vi "PositionSave_coMD.vi"() -> ()   [LabVIEW 2012]
doc: "SciScan 1.2 160622\n<b>Description</b>\n-------------\nThis is the Main VI for the Position Save Module and has a UI.\n\nThe module has a dependency with the main Sci-Scan software as it listens for events using the GFG."
uses:
  Custom Control and Typedefs/ChannelSelector_for_PosSave.ctl
  Custom Controls/PositionSaveMod.ctl
  Custom Control and Typedefs/Overlay Control.ctl
  SubVIs/PositionSaveFGVCommands.ctl
  Custom Control and Typedefs/UI Controls Refnum.ctl
  <vilib>/vision/Image Controls.llb/IMAQ Image.ctl
  Custom Control and Typedefs/ImageCluster.ctl
  SubVIs/Chnl_2_tab_Commands.ctl
  SubVIs/Image Validity FGV_Commands.ctl
  Custom Controls/MAIN Image panel tab Control type def.ctl
  CommonResource VIs/UI Control and Indicator properties_Commands.ctl
  CommonResource VIs/FormatTableStyle_Commands.ctl
  Custom Control and Typedefs/PositionData.ctl
  SubVIs/ImageIO_commands.ctl
  GFG/GFG library.lvlib
panel:
  in  "no of grid lines 2":dbl(slide)=2.0 caption="Grid" min=0.0 step=1.0 scale=0.0..20.0
  in  "FOCUS2":bool
  in  "Overlay Controls":T1={"auto scale\n      Red "=TRUE, "Min Max Saved (Green)"={0.0, 2047.0}, "auto scale\n      Blue"=TRUE, "Min Max Saved (Red)"={0.0, 2047.0}} {"Min Max Saved (Red)" scale=0.0..2047.0; "Min Max Saved (Green)" scale=0.0..2047.0}
  in  "Hide":T2
  in  "Copy Button":bool
  out "File Path":path
  in  "Overlay":bool
  in  "Table Navigation Cluster":T3
  in  "Vert_Cluster":T4
  in  "Big_Table":string[][](table)
  in  "Notes_Table":string[][](table)
  in  "Source":T5
  in  "step.size.z 2":u16(ring)=6 items=["  1"=1, "  2"=2, "  5"=5, " 10"=10, " 20"=20, " 50"=50, "100"=100]
  in  "Stage Stop 2":bool
  in  "Z UP 2":bool
  in  "Z DOWN 2":bool
  out "String 26":string
  in  "step.size.xy 2":u16(ring)=6 items=["  1"=1, "  2"=2, "  5"=5, " 10"=10, " 20"=20, " 50"=50, "100"=100]
  in  "Y UP 2":bool
  in  "X LEFT 2":bool
  in  "Y DOWN 2":bool
  in  "X RIGHT 2":bool
  out "String 25":string
  in  "setY 2":dbl caption="Z-Stepper" format="%#.1f"
  in  "setX 2":dbl caption="Z-Stepper" format="%#.1f"
  in  "setZ 2":dbl caption="set" format="%#.1f"
  out "String 24":string
  out "posZ 2":dbl caption="actual" format="%#.1f"
  out "posX 2":dbl caption="Z-Stepper" format="%#.1f"
  out "posY 2":dbl caption="Z-Stepper" format="%#.1f"
  out "String 23":string
  in  "Hor_Cluster":T6
  out "XY Graph":cluster{dbl[], dbl[]}[](graph)
  out "Saved Image":T7(plugin-control)
  out "Current Image":T7(plugin-control)
  # "abs  pos."
  # "x"
  # "y"
  # "z"
  # "pos."
  # "x"
  # "y"
  # "z"
  # "Red (Current Image)"
  # "Blue (Saved Image)"
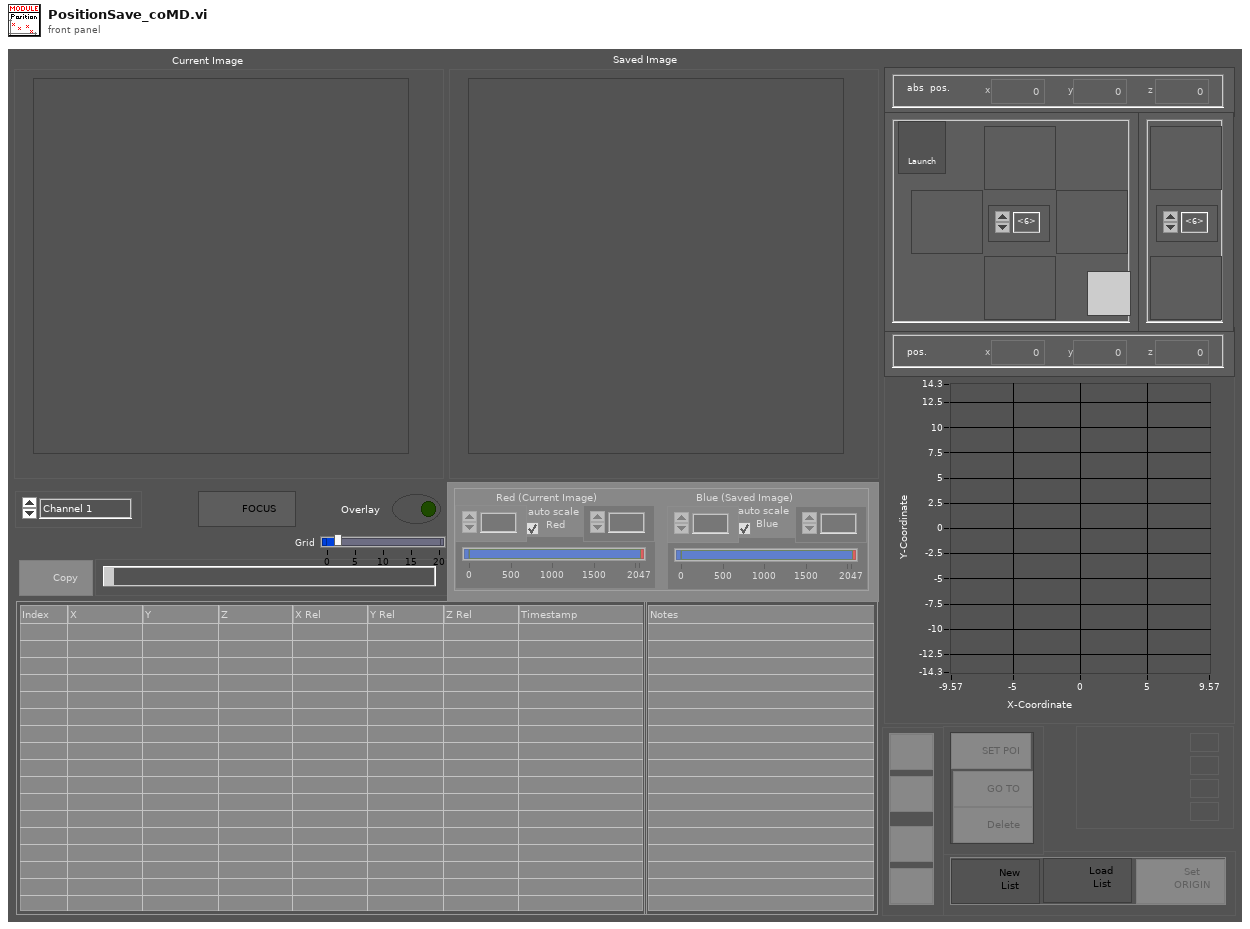
[diagram p1: front panel]
types:
  T1 = typedef "Overlay Control.ctl" = cluster{"auto scale\n      Red ":bool, "Min Max Saved (Green)":cluster{dbl, dbl}, "auto scale\n      Blue":bool, "Min Max Saved (Red)":cluster{dbl, dbl}}
  T2 = typedef "PositionSaveMod.ctl" = bool
  T3 = cluster{"Table Index Up":bool, "Table Index Up-End":bool, "Table Index Down":bool, "Table Index Down-End":bool}
  T4 = cluster{"Delete item":bool, "SET POI":bool, "GO TO":bool}
  T5 = typedef "ChannelSelector_for_PosSave.ctl" = enum16{"Channel 1", "Channel 2", "Channel 3", "Channel 4"}
  T6 = cluster{"New List":bool, "Load List":bool, "Set new Origin":bool}
  T7 = typedef "IMAQ Image.ctl" = refnum<image>
  T8 = typedef "Image Type" = u32
  T9 = typedef "UI Controls Refnum.ctl" = cluster{"GO TO":refnum<vi>, "Load List":refnum<vi>, "Big Table":refnum<vi>, "Notes Table":refnum<vi>, "New List":refnum<vi>, "Delete Item":refnum<vi>, "Set New Origin":refnum<vi>, "Set POI":refnum<vi>, "Saved Image":refnum<vi>, "Current Image":refnum<vi>, "step.size.xy 2":refnum<vi>, "step.size.z 2":refnum<vi>, "Source":refnum<vi>, "Table Up-End":refnum<vi>, "Table Up":refnum<vi>, "Table Down":refnum<vi>, "Table Down-End":refnum<vi>, "Copy Button":refnum<vi>, "Hide":refnum<vi>, "Overlay Controls":refnum<vi>, "Overlay":refnum<vi>, "XYGraph":refnum<vi>, "FOCUS2":refnum<vi>}
  T10 = typedef "PositionSaveFGVCommands.ctl" = enum16{"Initialize", "NewList", "LoadList", "CopyList", "DeleteSelected", "SetPosition", "SetNewOrigin", "UpdateEntireTable", "GetPosition", "Shutdown and Cleanup"}
  T11 = enum8{"Enabled", "Disabled", "Disabled and Grayed Out"}
  T12 = typedef "ImageCluster.ctl" = cluster{"CurrentImage":T7, "SavedImage":T7}
  T13 = enum32{"Invalid", "Standard", "Closed", "Hidden", "Minimized", "Maximized"}
  T14 = typedef "Image Validity FGV_Commands.ctl" = enum16{"Set validity status", "Get Validity status"}
  T15 = typedef "Chnl_2_tab_Commands.ctl" = enum16{"ChannelToTab", "TabToChannel"}
  T16 = typedef "MAIN Image panel tab Control type def.ctl" = enum32{"Channel 1", "Channel 2", "Channel 3", "Channel 4", "all channels", "RGB overlay", "ROI", "arbitrary line scan"}
  T17 = typedef "UI Control and Indicator properties_Commands.ctl" = enum16{"Enable", "Disable", "Disable and Grey", "Make Visible", "Make Invisible"}
  T18 = cluster{"moveXabs":dbl, "moveYabs":dbl, "moveZabs":dbl}
  T19 = typedef "FormatTableStyle_Commands.ctl" = enum16{"Colour Row", "Uncolour Row", "Bold Row", "Clear table", "UpdateVisibleRows", "Set Row Height", "Enabled Row style", "Disabled Row Style"}
  T20 = typedef "PositionData.ctl" = cluster{"X":dbl, "Y":dbl, "Z":dbl, "Base Path":path}
  T21 = typedef "ImageIO_commands.ctl" = enum16{"ReadImage", "WriteImage"}
  T22 = cluster{"WaveformChartRef":refnum<vi>, "DigitalRef":refnum<vi>, "ArrayRef":refnum<vi>, "TabControlRef":refnum<vi>, "EnumRef":refnum<vi>, "RingRef":refnum<vi>, "BooleanRef":refnum<vi>, "KnobRef":refnum<vi>, "SlideRef":refnum<vi>, "PathRef":refnum<vi>, "StringRef":refnum<vi>, "ComboBox":refnum<vi>, "WaveformGraphRef":refnum<vi>}
  T23 = typedef "LVRowAndColumnTypeDef.ctl" = cluster{"Row":i32, "Column":i32}
  T24 = typedef "eventvkey.ctl" = enum16{"ASCII", "Enter", "Return", "Shift", "Ctrl", "Alt", "Cmd", "Opt", "Caps", "NumLock", "Clear", "Break", "Up", "Down", "Left", "Right", "Insert", "Delete", "Home", "End", "PageUp", "PageDown", "Escape", "Help", "Pause", "ScrollLock", "F1", "F2", "F3", "F4", "F5", "F6", "F7", "F8", "F9", "F10", "F11", "F12", "F13", "F14", "F15", "F16", "F17", "F18", "F19", "F20", "F21", "F22", "F23", "F24", "Play", "VolumeUp", "VolumeDown", "Mute", "Two Byte Char"}
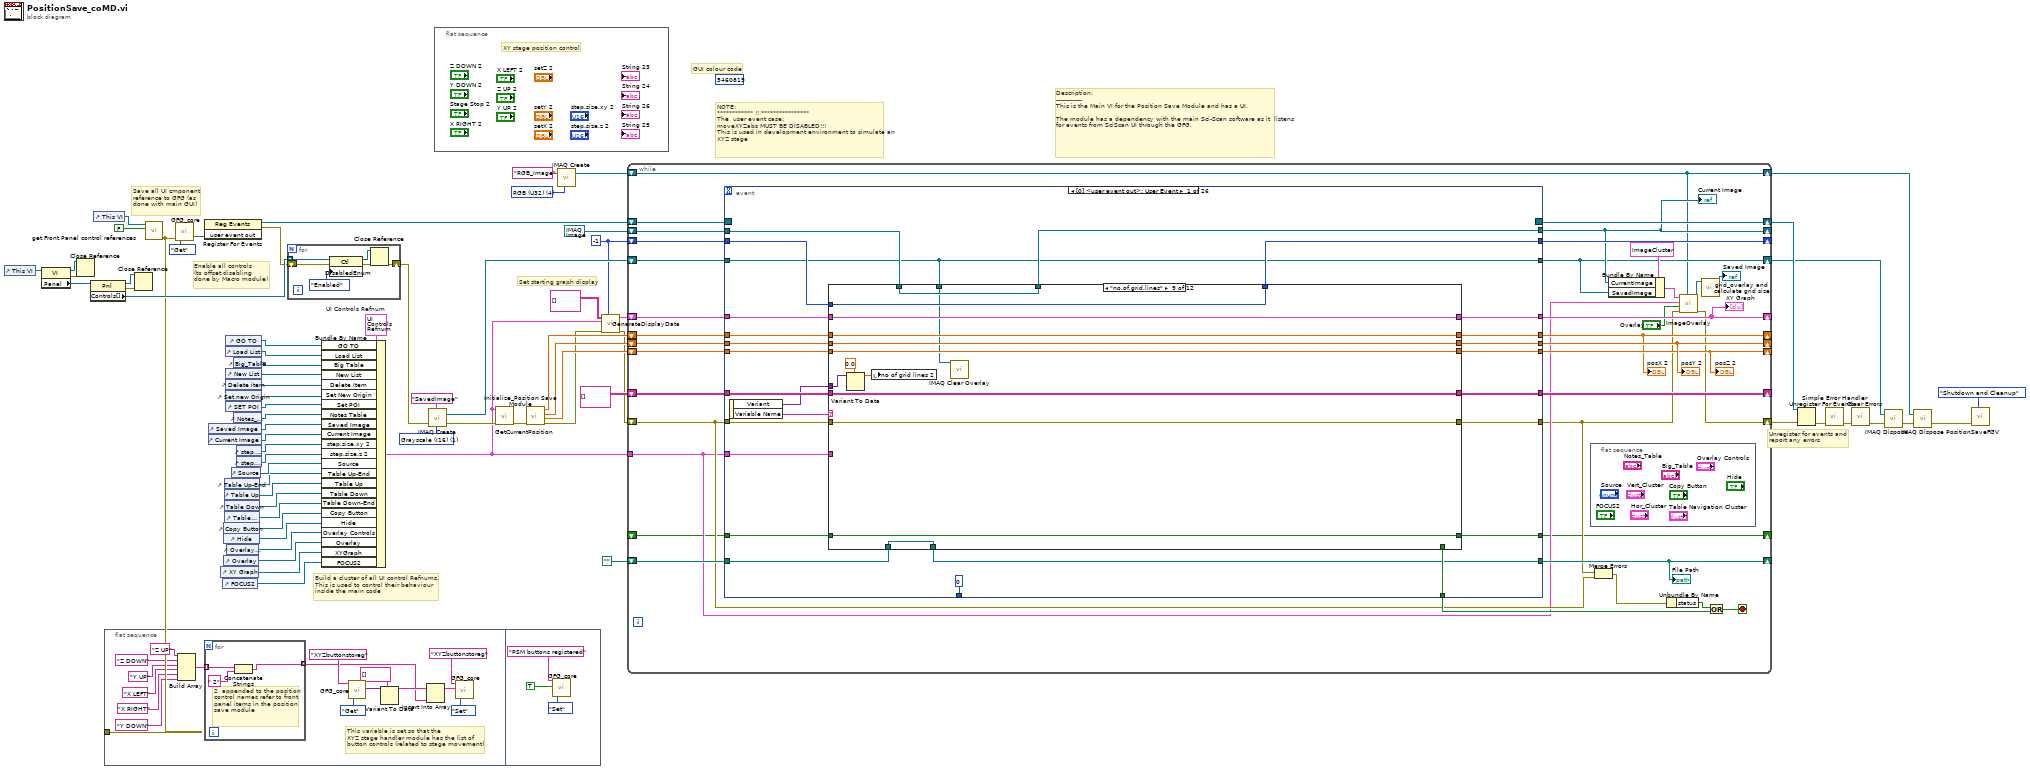
[diagram p0: block diagram]
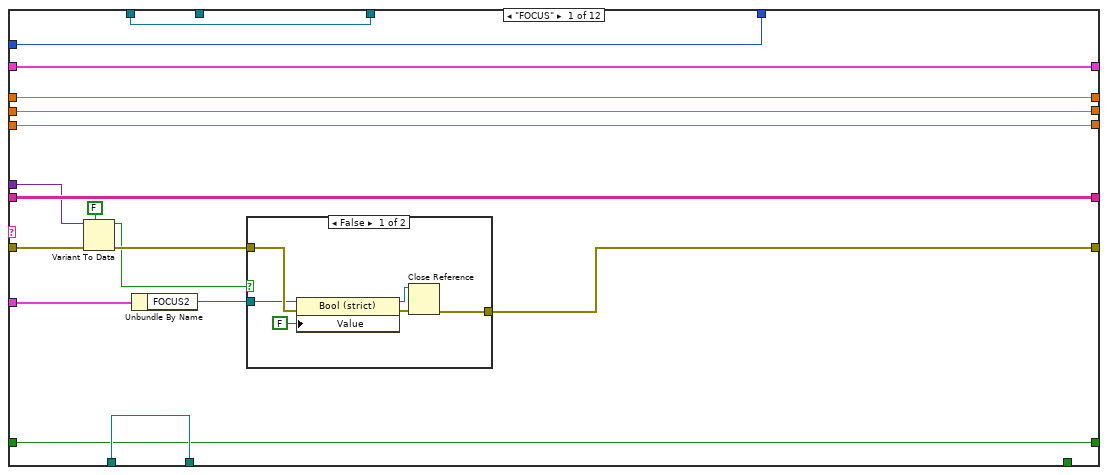
[diagram p2: hidden frame]
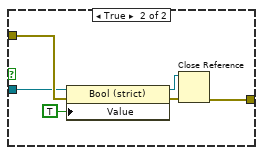
[diagram p3: hidden frame]
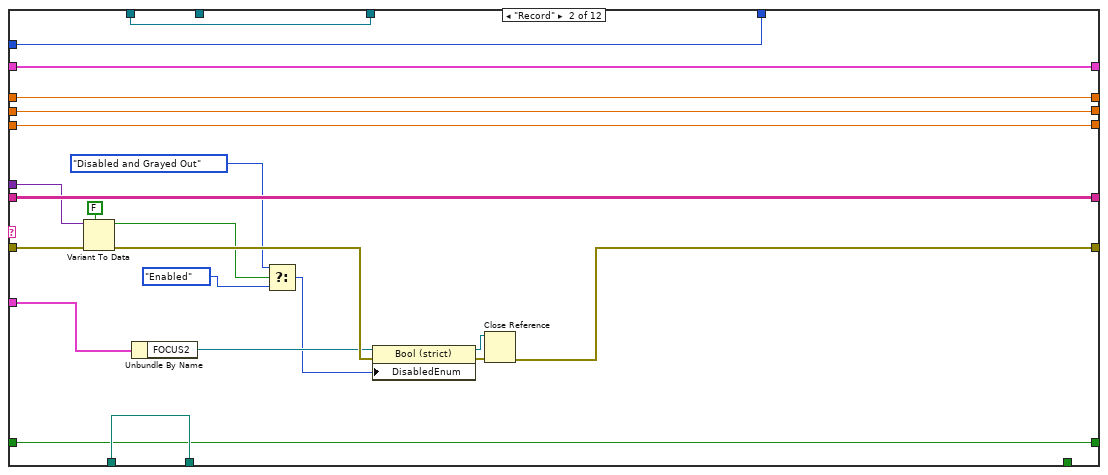
[diagram p4: hidden frame]
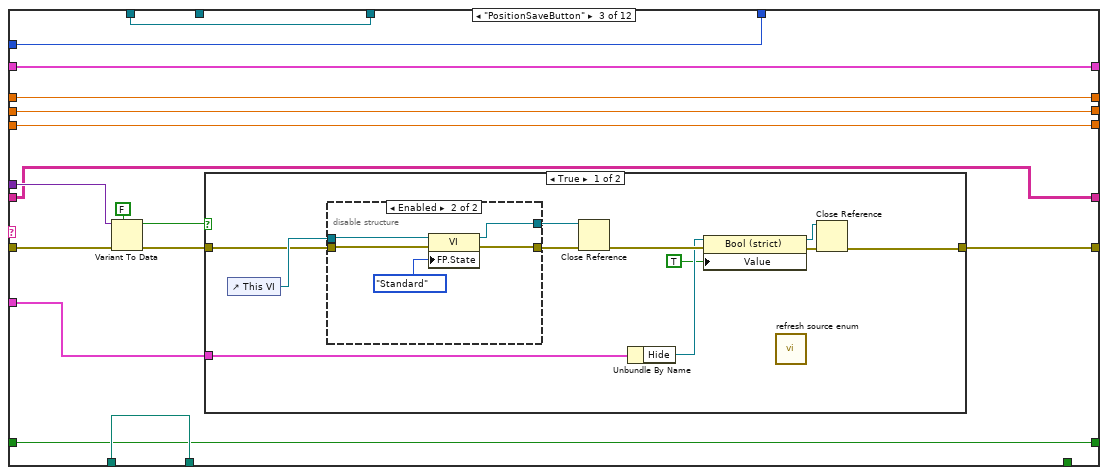
[diagram p5: hidden frame]
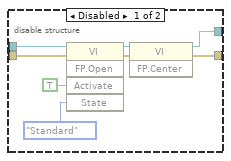
[diagram p6: hidden frame]
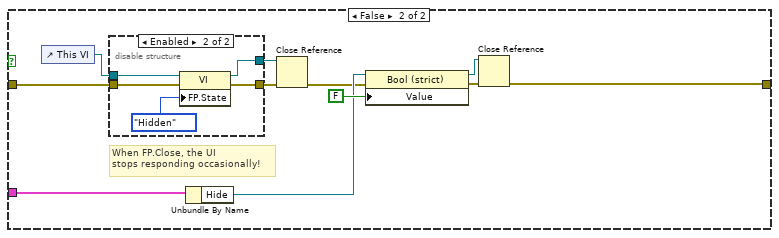
[diagram p7: hidden frame]
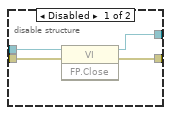
[diagram p8: hidden frame]
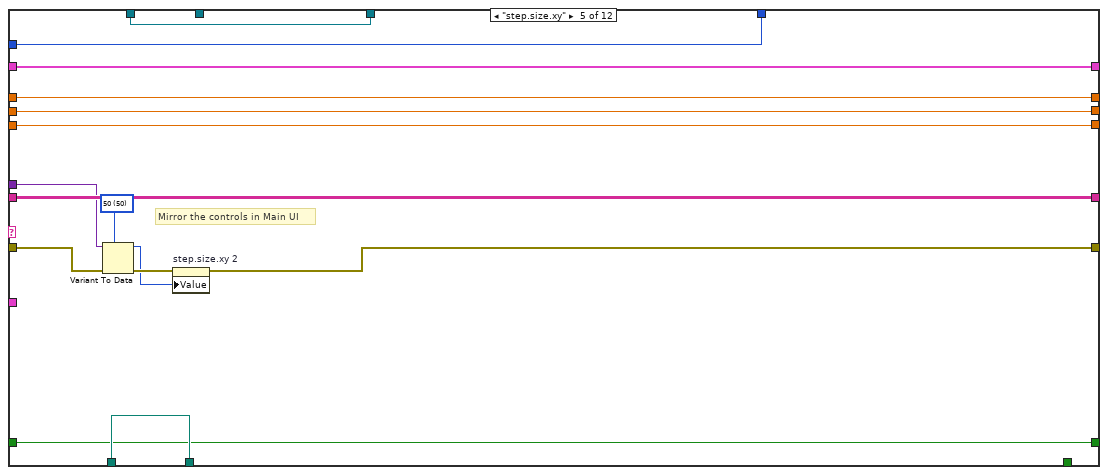
[diagram p10: hidden frame]
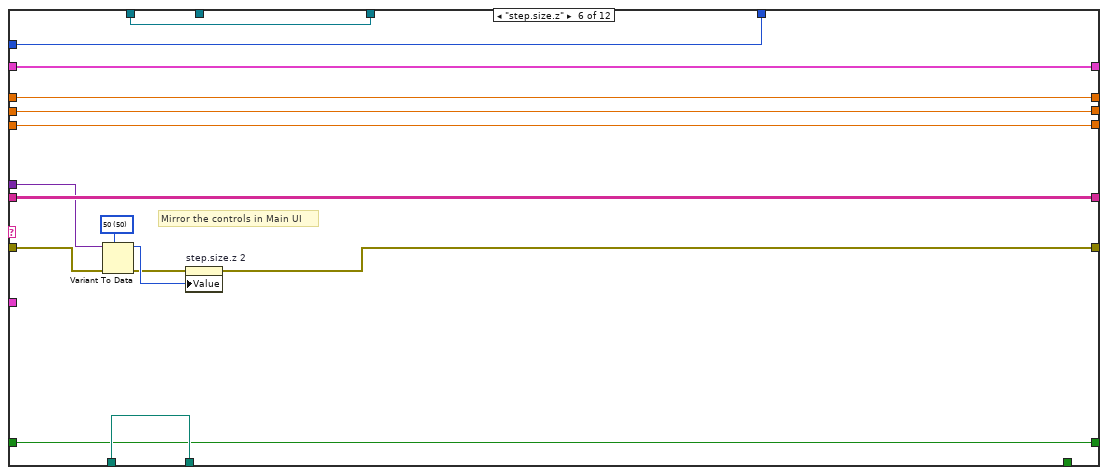
[diagram p11: hidden frame]
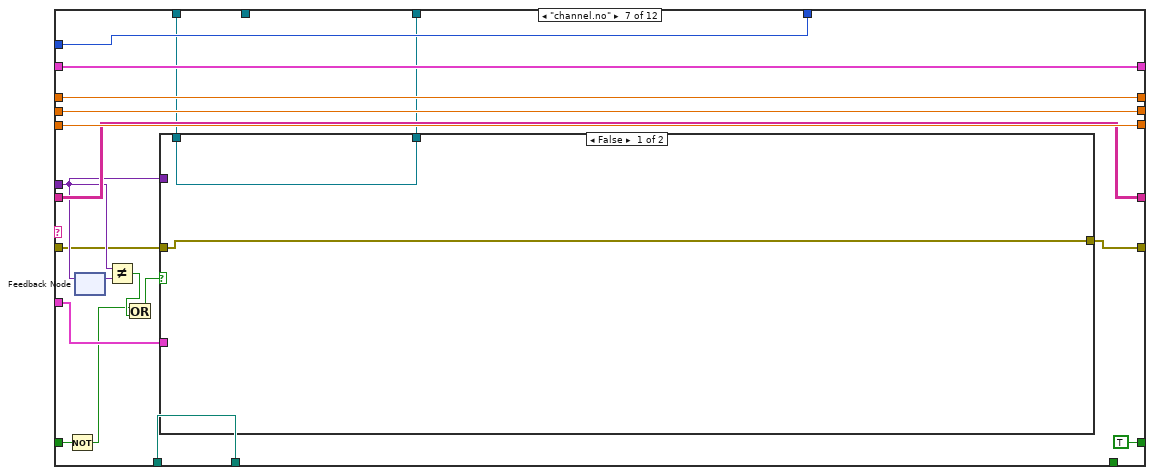
[diagram p12: hidden frame]
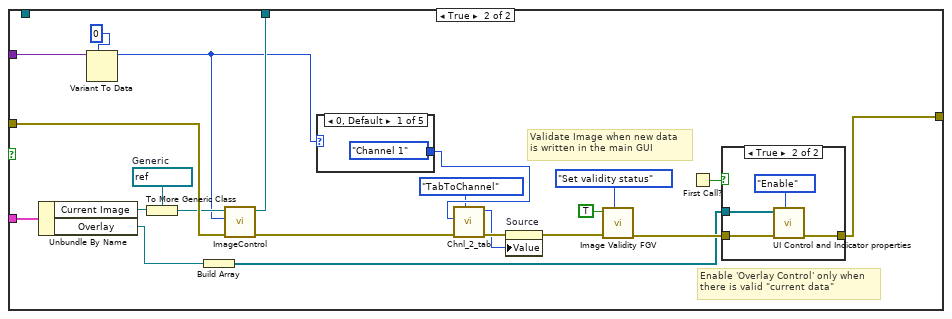
[diagram p13: hidden frame]
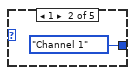
[diagram p14: hidden frame]
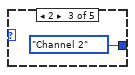
[diagram p15: hidden frame]
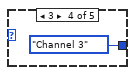
[diagram p16: hidden frame]
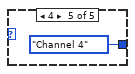
[diagram p17: hidden frame]
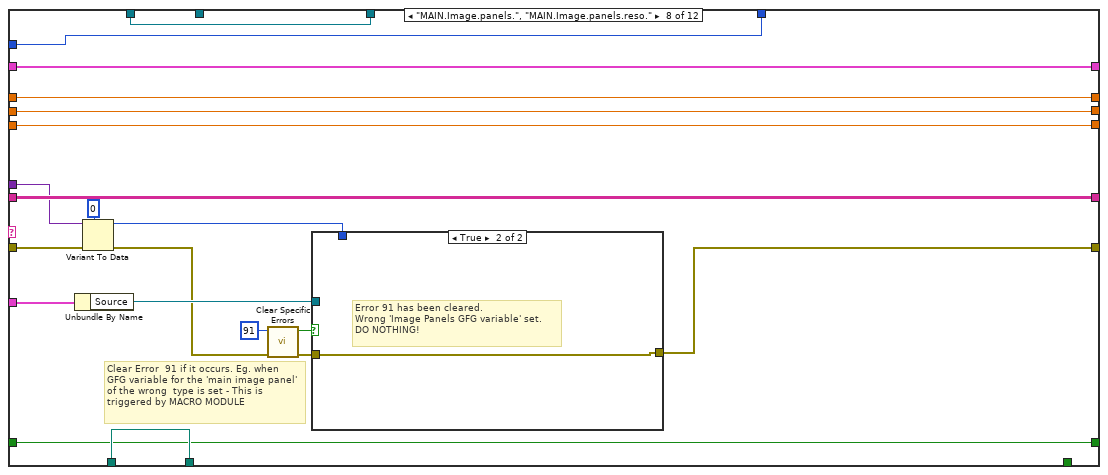
[diagram p19: hidden frame]
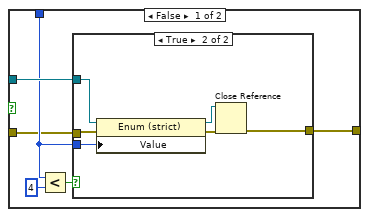
[diagram p20: hidden frame]
diagram:
  w26 = T8 4 items=["Grayscale (U8)", "Grayscale (I16)", "Grayscale (SGL)", "Complex (CSG)", "RGB (U32)", "HSL (U32)", "RGB (U64)", "Grayscale (U16)"] ("Image Type")
  w37 = T8 1 items=["Grayscale (U8)", "Grayscale (I16)", "Grayscale (SGL)", "Complex (CSG)", "RGB (U32)", "HSL (U32)", "RGB (U64)", "Grayscale (U16)"] ("Image Type")
  (unwired) u32 5460819 ("Active Cell:Cell Background Color")
  w18 = -1
  w61 = T9 {"GO TO"=refnum, "Load List"=refnum, "Big Table"=refnum, "Notes Table"=refnum, "New List"=refnum, "Delete Item"=refnum, "Set New Origin"=refnum, "Set POI"=refnum, "Saved Image"=refnum, "Current Image"=refnum, "step.size.xy 2"=refnum, "step.size.z 2"=refnum, "Source"=refnum, "Table Up-End"=refnum, "Table Up"=refnum, "Table Down"=refnum, "Table Down-End"=refnum, "Copy Button"=refnum, "Hide"=refnum, "Overlay Controls"=refnum, "Overlay"=refnum, "XYGraph"=refnum, "FOCUS2"=refnum}  # UI Controls Refnum
  # "Enable all controls\n(to offset disabling \ndone by Macro module)"
  # "Set starting graph display"
  # "GUI colour code"
  # "Save all UI cmponent reference to GFG (as done with main GUI)"
  # "NOTE:\n************ !! ****************\nThe  user event case:\nmoveXYZabs MUST BE DISABLED!!!\nThis is used in development environment to simulate an XYZ stage"
  # "Build a cluster of all UI control Refnums.\nThis is used to control their behaviour \ninside the main code"
  # "Unregister for events and \nreport any errors"
  # "Description:\n-------------\nThis is the Main VI for the Position Save Module and has a UI.\n\nThe module has a dependency with the main Sci-Scan software as it  listens for events from SciScan UI through the GFG."
  n1 = control-ref of="This VI"() -> (w10:refnum<vi>)
  n2 = property class="VI"(reference=w10) -> (reference out=w7:refnum<vi>, error out=w8:errorcluster, "Panel"=w9:refnum<vi>)  [unwired: 1 in]
  n3 = Close Reference(reference=w7, error in (no error)=w8) -> ()  [unwired: 1 out]
  n4 = property class="Pnl"(reference=w9) -> (reference out=w5:refnum<vi>, error out=w6:errorcluster, "Controls[]"=w4:refnum<vi>[])  [unwired: 1 in]
  n5 = control-ref of="This VI"() -> (w54:refnum<vi>)
  n6 = flat-sequence {
    tunnel: w1 -> [_]
    frame #0 {
      # "This variable is set so that the \nXYZ stage handler module has the list of\nbutton controls (related to stage movement)"
      n7 = Build Array("Z UP" ("Variable Name in"), "Z DOWN" ("Variable Name in"), "Y UP" ("Variable Name in"), "X LEFT" ("Variable Name in"), "X RIGHT" ("Variable Name in"), "Y DOWN" ("Variable Name in")) -> (w79:string[])
      n8 = for {
        tunnel: w79 -> [w88] mode=indexing
        tunnel: [w86] -> w70 mode=indexing
        # "2  appended to the position control names refer to front panel items in the position save module"
        n9 = Concatenate Strings(w88, " 2" ("string")) -> (w86:string)
      }
      n10 = call "GFG_core.vi"("Variable Name in"="XYZbuttonstoreg", "Action"=enum16{"Init", "Set", "Get"}."Get") -> ("Variant Out"=w73:variant)  [unwired: 11 in, 6 out]
      n11 = Variant To Data(type=string[] [], Variant=w73) -> (data=w71:string[])  [unwired: 1 in, 1 out]
      n12 = Insert Into Array(array=w71, new element=w70) -> (w72:string[])  [unwired: 1 in]
      n13 = call "GFG_core.vi"("Variable Name in"="XYZbuttonstoreg", "Variant in"=w72, "Action"=enum16{"Init", "Set", "Get"}."Set") -> ()  [unwired: 10 in, 7 out]
    }
    frame #1 {
      n14 = call "GFG_core.vi"("Variable Name in"="PSM buttons registered", "Variant in"=TRUE, "Action"=enum16{"Init", "Set", "Get"}."Set") -> ()  [unwired: 10 in, 7 out]
    }
  }
  n15 = Close Reference(reference=w5, error in (no error)=w6) -> ()  [unwired: 1 out]
  n16 = call "get Front Panel control references.vi"("Signalling (Default: T)"=FALSE, "Main VI"=w54) -> ("error out"=w1:errorcluster)  [unwired: 9 in]
  n17 = call "GFG_core.vi"("error in (no error)"=w1, "Action"=enum16{"Init", "Set", "Get"}."Get") -> ("user event out"=w67:refnum<user-event>)  [unwired: 11 in, 6 out]
  n18 = register-events(w67) -> (reference out=w68:refnum<event-registration>, error out=w3:errorcluster)  [unwired: 2 in]
  n19 = control-ref of="Saved Image"() -> (w50:refnum<vi>)
  n20 = control-ref of="Current Image"() -> (w49:refnum<vi>)
  n21 = control-ref of="XY Graph"() -> (w22:refnum<vi>)
  n22 = control-ref of="FOCUS2"() -> (w17:refnum<vi>)
  n23 = control-ref of="Overlay"() -> (w23:refnum<vi>)
  n24 = control-ref of="Copy Button"() -> (w35:refnum<vi>)
  n25 = control-ref of="Hide"() -> (w31:refnum<vi>)
  n26 = control-ref of="Table Up-End"() -> (w44:refnum<vi>)
  n27 = control-ref of="Table Up"() -> (w43:refnum<vi>)
  n28 = control-ref of="Table Down"() -> (w42:refnum<vi>)
  n29 = control-ref of="Table Down-End"() -> (w41:refnum<vi>)
  n30 = control-ref of="GO TO"() -> (w60:refnum<vi>)
  n31 = control-ref of="Load List"() -> (w59:refnum<vi>)
  n32 = control-ref of="New List"() -> (w58:refnum<vi>)
  n33 = control-ref of="Delete item"() -> (w57:refnum<vi>)
  n34 = control-ref of="Set new Origin"() -> (w56:refnum<vi>)
  n35 = control-ref of="SET POI"() -> (w55:refnum<vi>)
  n36 = control-ref of="Overlay Controls"() -> (w28:refnum<vi>)
  n37 = control-ref of="Source"() -> (w46:refnum<vi>)
  n38 = control-ref of="Big_Table"() -> (w40:refnum<vi>)
  n39 = control-ref of="Notes_Table"() -> (w52:refnum<vi>)
  n40 = control-ref of="step.size.xy 2"() -> (w48:refnum<vi>)
  n41 = control-ref of="step.size.z 2"() -> (w47:refnum<vi>)
  n42 = for {
    tunnel: w4 -> [w97] mode=indexing
    shift-right: [w93] -> w2
    shift-left: w3 -> [w92]
    n43 = property class="Ctl"(reference=w97, error in=w92, "DisabledEnum"=T11."Enabled" ("Disabled")) -> (reference out=w94:refnum<vi>, error out=w95:errorcluster)
    n44 = Close Reference(reference=w94, error in (no error)=w95) -> (error out=w93:errorcluster)
  }
  n45 = Bundle By Name(cluster=w61, "GO TO"=w60, "Load List"=w59, "Big Table"=w40, "New List"=w58, "Delete Item"=w57, "Set New Origin"=w56, "Set POI"=w55, "Notes Table"=w52, "Saved Image"=w50, "Current Image"=w49, "step.size.xy 2"=w48, "step.size.z 2"=w47, "Source"=w46, "Table Up-End"=w44, "Table Up"=w43, "Table Down"=w42, "Table Down-End"=w41, "Copy Button"=w35, "Hide"=w31, "Overlay Controls"=w28, "Overlay"=w23, "XYGraph"=w22, "FOCUS2"=w17) -> (w21:T9)
  n46 = call "IMAQ Create"("Image Name"="SavedImage", "Image Type"=w37, "error in (no error)"=w2) -> ("New Image"=w36:T7, "error out"=w38:errorcluster)  [unwired: 2 in]
  n47 = flat-sequence {
    frame #0 {
      # "XY stage position control"
    }
  }
  n48 = call "Initialize_Position Save Module.vi"("Error In"=w38, "UI Controls Refnum"=w21) -> ("Error Out"=w45:errorcluster)  [unwired: 9 in]
  n49 = call "GetCurrentPosition.vi"("Error In"=w45) -> ("Error Out"=w20:errorcluster, "Z"=w64:dbl, "Y"=w65:dbl, "X"=w66:dbl)  [unwired: 7 in]
  n50 = call "IMAQ Create"("Image Name"="RGB_Image", "Image Type"=w26) -> ("New Image"=w25:T7)  [unwired: 3 in, 1 out]
  n51 = call "GenerateDisplayData.vi"("Index"=w18, "Error In"=w20, "UI Controls Refnum"=w21, "2D Data IN"=string[][] []) -> ("Error Out"=w19:errorcluster, "Plot Data OUT"=w29:cluster{dbl[], dbl[]}[])  [unwired: 4 in, 2 out]
  n52 = while {
    shift-right: [w102] -> w33
    shift-left: w19 -> [w112]
    shift-right: [w129] -> w62
    shift-left: w68 -> [w130]
    shift-right: [w114] -> _
    shift-left: w66 -> [w128]
    shift-right: [w123] -> _
    shift-left: w65 -> [w127]
    shift-right: [w122] -> _
    shift-left: w64 -> [w126]
    shift-right: [w113] -> _
    shift-left: w29 -> [w125]
    shift-right: [w120] -> _
    shift-left: string[][] [] ("Formatted Table Data") -> [w124]
    tunnel: w21 -> [w110]
    shift-right: [w108] -> _
    shift-left: T7 refnum ("Saved Image OUT") -> [w121]
    shift-right: [w118] -> _
    shift-left: w18 -> [w119]
    shift-right: [w107] -> w13
    shift-left: w36 -> [w117]
    shift-right: [w115] -> _
    shift-left: path "" -> [w116]
    shift-right: [w105] -> w12
    shift-left: w25 -> [w105]
    shift-right: [w101] -> _
    shift-left: _ -> [w100]
    stop <- w131 stop-if-true
    n53 = event shown="[0] <user event out>: User Event" {
      selector: w130 -> [_ _ _ _ w596 w676 w743 w869 w951 w1060 _ _ w1268 w1299 _ _ _ _ _ _ _ _ _ _ _ _]
      dyn-events: [_ _ _ _ w589 w670 w738 w867 w946 w1056 _ _ w1263 w1291 _ _ _ _ _ _ _ _ _ _ _ _] -> w129
      timeout: _ -> [_ _ _ _ _ _ _ _ _ _ _ _ _ _ _ _ _ _ _ _ _ _ _ _ _ _]
      tunnel: [w159 _ _ _ _ _ _ _ _ _ _ _ _ _ _ _ _ _ _ _ _ _ _ _ FALSE _] -> w133
      tunnel: w128 -> [w155 w543 w559 w581 w588 w669 w771 w866 w945 w1054 w1183 w1235 w1262 w1294 w1372 w1421 w1471 w1516 w1564 w1595 w1615 w1635 w1696 w1713 w1720 w1766]
      tunnel: w127 -> [w154 w542 w558 w580 w587 w668 w770 w865 w944 w1053 w1182 w1234 w1261 w1293 w1371 w1420 w1470 w1515 w1563 w1594 w1614 w1634 w1695 w1712 w1719 w1765]
      tunnel: w126 -> [w153 w541 w557 w579 w586 w667 w760 w864 w943 w1052 w1181 w1233 w1260 w1292 w1370 w1419 w1469 w1514 w1562 w1593 w1613 w1633 w1694 w1711 w1718 w1764]
      tunnel: [w156 w543 w559 w581 w585 w666 w734 w863 w942 w1051 w1183 w1235 w1259 w1290 w1372 w1421 w1471 w1516 w1564 w1595 w1615 w1635 w1696 w1713 w1720 w1766] -> w114
      tunnel: [w157 w542 w558 w580 w584 w665 w733 w862 w941 w1050 w1182 w1234 w1258 w1288 w1371 w1420 w1470 w1515 w1563 w1594 w1614 w1634 w1695 w1712 w1719 w1765] -> w123
      tunnel: [w158 w541 w557 w579 w583 w664 w732 w861 w940 w1049 w1181 w1233 w1257 w1287 w1370 w1419 w1469 w1514 w1562 w1593 w1613 w1633 w1694 w1711 w1718 w1764] -> w122
      tunnel: [w144 w540 w556 w578 w606 w682 w765 w889 w956 w1075 w1157 w1207 w1284 w1319 w1348 w1397 w1449 w1496 w1561 w1592 w1612 w1618 w1693 w1710 w1717 w1763] -> w113
      tunnel: w125 -> [w145 w540 w556 w578 _ _ w766 w888 _ w1074 _ _ w1284 w1319 _ _ _ _ w1561 w1592 w1612 _ w1693 w1710 w1717 w1763]
      tunnel: [w151 w535 w552 w574 w608 w683 w769 w890 w959 w1078 w1158 w1208 w1277 w1317 w1351 w1399 w1451 w1498 w1560 w1588 w1611 w1622 w1689 w1706 w1721 w1758] -> w120
      tunnel: w112 -> [w152 w521 w547 w572 w597 w677 w745 w871 w953 w1062 w1179 w1231 w1271 w1300 w1365 w1414 w1466 w1509 w1558 w1587 w1601 w1627 w1673 w1705 w1723 w1757]
      tunnel: [w150 w520 w546 w572 w592 w672 w739 w872 w948 w1057 w1155 w1209 w1264 w1289 w1350 w1401 w1453 w1500 w1544 w1586 w1598 w1619 w1672 w1704 w1727 w1757] -> w103
      tunnel: w124 -> [w149 w535 w552 w574 w621 w692 w756 w885 w971 w1079 w1158 w1208 w1277 w1315 w1351 w1399 w1451 w1498 w1560 w1588 w1611 w1622 w1689 w1706 w1721 w1758]
      tunnel: w110 -> [w146 _ w549 _ w599 w680 w751 w886 w957 w1076 w1154 w1206 w1282 w1304 w1349 w1398 w1450 w1497 _ _ _ w1621 _ _ _ _]
      tunnel: [w143 w539 w555 w577 w618 w689 w762 w881 w974 w1070 w1163 w1216 w1283 w1318 w1357 w1406 w1447 w1505 w1555 w1584 w1610 w1629 w1692 w1702 w1725 w1762] -> w108
      tunnel: w121 -> [w139 w539 w555 w577 w618 w689 w762 w881 w974 w1070 w1163 w1216 w1283 w1318 w1357 w1406 w1447 w1505 w1555 w1584 w1610 w1629 w1692 w1702 w1725 w1762]
      tunnel: w119 -> [w147 w538 w554 w576 w620 w691 w768 w884 w977 w1073 w1176 w1228 w1276 w1303 w1362 w1413 w1465 w1508 w1554 w1583 w1609 w1626 w1686 w1701 w1724 w1761]
      tunnel: [w140 w538 w554 w576 w607 w681 w767 w883 w958 w1077 w1156 w1211 w1276 w1303 w1353 w1400 w1452 w1499 w1554 w1583 w1609 w1620 w1686 w1701 w1724 w1761] -> w118
      tunnel: [w134 w537 w553 w575 w615 w687 w748 w878 w976 w1068 w1161 w1214 w1275 w1311 w1355 w1404 w1448 w1503 w1553 w1582 w1608 w1624 w1691 w1700 w1726 w1752] -> w107
      tunnel: w117 -> [w134 w537 w553 w575 w617 w690 w763 w880 w973 w1071 w1164 w1217 w1275 w1311 w1358 w1407 w1457 w1506 w1553 w1582 w1608 w1625 w1691 w1700 w1726 w1760]
      tunnel: [w141 w534 w551 w573 w614 w685 w750 w877 w967 w1066 w1160 w1213 w1274 w1310 w1354 w1403 w1455 w1502 w1549 w1581 w1607 w1632 w1690 w1699 w1716 w1756] -> w115
      tunnel: w116 -> [w142 w534 w551 w573 _ _ w749 _ w966 w1065 w1160 w1213 w1274 w1310 w1354 w1403 w1455 w1502 w1549 w1581 w1607 w1632 w1690 w1699 w1716 w1756]
      tunnel: [0 ("x-y 2") _ 1 ("x-y 2") 2 ("x-y 2") 3 ("x-y 2") 4 ("x-y 2") 5 ("x-y 2") 6 ("x-y 2") 7 ("x-y 2") 8 ("x-y 2") 9 ("x-y 2") 10 ("x-y 2") 11 ("x-y 2") 12 ("x-y 2") 13 ("x-y 2") 14 ("x-y 2") 15 ("x-y 2") 16 ("x-y 2") 17 ("x-y 2") 18 ("x-y 2") 19 ("x-y 2") 20 ("x-y 2") 21 ("x-y 2") 22 ("x-y 2") 23 ("x-y 2") _] -> _
      tunnel: [w136 w519 w544 w570 w582 w663 w731 w860 w939 w1048 w1152 w1204 w1256 w1286 w1346 w1395 w1445 w1494 w1539 w1579 w1596 w1616 w1671 w1697 w1714 w1759] -> w101
      tunnel: w100 -> [w135 w519 w544 w570 w582 w663 w731 w860 w939 w1048 w1152 w1204 w1256 w1286 w1346 w1395 w1445 w1494 w1539 w1579 w1596 w1616 w1671 w1697 w1714 w1759]
      event User Event {
        n54 = event-data() -> ("Variant"=w148:variant, "Variable Name"=w137:string)  [unwired: 1 in]
        n55 = case shown="\"no.of.grid.lines\"" w137 {
          tunnel: [_ _ _ _ _ _ _ _ _ _ _ w465] -> w159
          tunnel: [w174 w208 w224 w274 w293 w308 w327 w381 w404 w421 w457 w492] -> w158
          tunnel: [w175 w209 w225 w275 w294 w309 w328 w382 w405 w422 w456 w492] -> w157
          tunnel: [w176 w210 w226 w276 w295 w310 w329 w383 w406 w423 w455 w492] -> w156
          tunnel: w155 -> [w176 w210 w226 w276 w295 w310 w329 w383 w406 w423 _ _]
          tunnel: w154 -> [w175 w209 w225 w275 w294 w309 w328 w382 w405 w422 _ _]
          tunnel: w153 -> [w174 w208 w224 w274 w293 w308 w327 w381 w404 w421 _ _]
          tunnel: w152 -> [w167 w201 w223 w272 w290 w305 w320 w374 w402 w417 w454 w489]
          tunnel: [w173 w207 w217 w273 w292 w307 w326 w380 w403 w418 w452 w486] -> w151
          tunnel: [w163 w198 w218 w272 w287 w302 w317 w371 w402 w419 w453 w464] -> w150
          tunnel: w149 -> [w173 w207 w217 w273 w292 w307 w326 w380 w403 w418 w452 _]
          tunnel: w148 -> [w165 w199 w221 _ w286 w301 w322 w379 w401 w420 _ _]
          tunnel: [w169 w203 w212 w280 w282 w297 w319 w375 w411 w413 w448 w472] -> w143
          tunnel: w147 -> [w170 w204 w214 w277 w283 w298 w323 w376 w407 w414 w447 w491]
          tunnel: w146 -> [w162 w197 w213 _ _ _ w318 w373 _ _ w449 w490]
          tunnel: w145 -> [w172 w206 w215 w279 w285 w300 w325 w378 w410 w416 _ _]
          tunnel: [w172 w206 w215 w279 w285 w300 w325 w378 w410 w416 w451 cluster{dbl[], dbl[]}[] [] ("Plot Data OUT")] -> w144
          tunnel: w142 -> [w171 w205 w216 w278 w284 w299 w324 w377 w409 w415 w450 _]
          tunnel: [w171 w205 w216 w278 w284 w299 w324 w377 w409 w415 w450 path ""] -> w141
          tunnel: [w170 w204 w214 w277 w283 w298 w323 w376 w407 w414 w447 0 ("Row")] -> w140
          tunnel: w139 -> [w169 w203 w212 w280 w282 w297 w311 w375 w411 w413 w448 w472]
          tunnel: [w160 w195 w211 w271 w281 w296 TRUE ("Validity status IN") w364 w408 w412 FALSE ("Validity status IN") w458] -> w136
          tunnel: w135 -> [w160 w195 w211 w271 w281 w296 w313 w364 w408 w412 _ w458]
          tunnel: w134 -> [_ _ _ _ _ _ _ _ w398 _ _ _]
          frame "FOCUS" {
            n56 = Variant To Data(error in=w167, type=FALSE ("Value"), Variant=w165) -> (data=w164:bool, error out=w166:errorcluster)
            n57 = Unbundle By Name(w162) -> ("FOCUS2"=w161:refnum<vi>)
            n58 = case shown="False" w164 {
              tunnel: w166 -> [w181 w187]
              tunnel: [w178 w184] -> w163
              tunnel: w161 -> [w177 w183]
              frame False {
                n59 = property class="Bool (strict)"(reference=w177, error in=w181, "Value"=FALSE) -> (reference out=w179:refnum<vi>, error out=w180:errorcluster)
                n60 = Close Reference(reference=w179, error in (no error)=w180) -> (error out=w178:errorcluster)
              }
              frame True {
                n61 = property class="Bool (strict)"(reference=w183, error in=w187, "Value"=TRUE) -> (reference out=w185:refnum<vi>, error out=w186:errorcluster)
                n62 = Close Reference(reference=w185, error in (no error)=w186) -> (error out=w184:errorcluster)
              }
            }
          }
          frame "Record" {
            n63 = Variant To Data(error in=w201, type=FALSE ("Value"), Variant=w199) -> (data=w194:bool, error out=w200:errorcluster)
            n64 = Unbundle By Name(w197) -> ("FOCUS2"=w196:refnum<vi>)
            n65 = Select(t=T11."Disabled and Grayed Out" ("Disabled"), s=w194, f=T11."Enabled" ("Disabled")) -> (s? t:f=w189:T11)
            n66 = property class="Bool (strict)"(reference=w196, error in=w200, "DisabledEnum"=w189) -> (reference out=w192:refnum<vi>, error out=w193:errorcluster)
            n67 = Close Reference(reference=w192, error in (no error)=w193) -> (error out=w198:errorcluster)
          }
          frame "PositionSaveButton" {
            n68 = Variant To Data(error in=w223, type=FALSE, Variant=w221) -> (data=w219:bool, error out=w220:errorcluster)
            n69 = case shown="True" w219 {
              tunnel: w220 -> [w236 w260]
              tunnel: [w227 w254] -> w218
              tunnel: w213 -> [w232 w253]
              frame True {
                n70 = control-ref of="This VI"() -> (w237:refnum<vi>)
                n71 = disable-structure shown="Enabled" {
                  disable-tunnel: w237 -> [w245 w249]
                  disable-tunnel: w236 -> [w244 w248]
                  disable-tunnel: [w239 w247] -> w235
                  disable-tunnel: [w238 w246] -> w234
                  frame Disabled {
                    n72 = invoke class="VI" method="FP.Open"(reference=w245, error in=w244, "Activate"=TRUE ("Activate?"), "State"=T13."Standard") -> (reference out=w241:refnum<vi>, error out=w240:errorcluster)  [unwired: 1 in, 3 out]
                    n73 = invoke class="VI" method="FP.Center"(reference=w241, error in=w240) -> (reference out=w238:refnum<vi>, error out=w239:errorcluster)  [unwired: 1 in, 1 out]
                  }
                  frame Enabled {
                    n74 = property class="VI"(reference=w249, error in=w248, "FP.State"=T13."Standard" ("Front Panel Window:State")) -> (reference out=w246:refnum<vi>, error out=w247:errorcluster)
                  }
                }
                n75 = Close Reference(reference=w234, error in (no error)=w235) -> (error out=w233:errorcluster)
                n76 = Unbundle By Name(w232) -> ("Hide"=w231:refnum<vi>)
                n77 = property class="Bool (strict)"(reference=w231, error in=w233, "Value"=T2 TRUE) -> (reference out=w228:refnum<vi>, error out=w229:errorcluster)
                n78 = call "refresh source enum.vi"() -> ()  [unwired: 12 in]
                n79 = Close Reference(reference=w228, error in (no error)=w229) -> (error out=w227:errorcluster)
              }
              frame False {
                # "When FP.Close, the UI\nstops responding occasionally!"
                n80 = control-ref of="This VI"() -> (w261:refnum<vi>)
                n81 = disable-structure shown="Enabled" {
                  disable-tunnel: w261 -> [w265 w268]
                  disable-tunnel: w260 -> [w264 w269]
                  disable-tunnel: [w263 w270] -> w259
                  disable-tunnel: [w262 w266] -> w258
                  frame Disabled {
                    n82 = invoke class="VI" method="FP.Close"(reference=w265, error in=w264) -> (reference out=w262:refnum<vi>, error out=w263:errorcluster)  [unwired: 1 in, 1 out]
                  }
                  frame Enabled {
                    n83 = property class="VI"(reference=w268, error in=w269, "FP.State"=T13."Hidden" ("Front Panel Window:State")) -> (reference out=w266:refnum<vi>, error out=w270:errorcluster)
                  }
                }
                n84 = Unbundle By Name(w253) -> ("Hide"=w252:refnum<vi>)
                n85 = Close Reference(reference=w258, error in (no error)=w259) -> (error out=w251:errorcluster)
                n86 = property class="Bool (strict)"(reference=w252, error in=w251, "Value"=T2 FALSE) -> (reference out=w255:refnum<vi>, error out=w256:errorcluster)
                n87 = Close Reference(reference=w255, error in (no error)=w256) -> (error out=w254:errorcluster)
              }
            }
          }
          frame Default {
          }
          frame "step.size.xy" {
            w291 = u16 50 items=["  1"=1, "  2"=2, "  5"=5, " 10"=10, " 20"=20, " 50"=50, "100"=100] ("step.size.xy 2")
            # "Mirror the controls in Main UI"
            n88 = Variant To Data(error in=w290, type=w291, Variant=w286) -> (data=w288:u16, error out=w289:errorcluster)
            n89 = property on="step.size.xy 2" class="Ring (strict)"(error in=w289, "Value"=w288) -> (error out=w287:errorcluster)  [unwired: 1 in, 1 out]
          }
          frame "step.size.z" {
            w306 = u16 50 items=["  1"=1, "  2"=2, "  5"=5, " 10"=10, " 20"=20, " 50"=50, "100"=100] ("step.size.xy 2")
            # "Mirror the controls in Main UI"
            n90 = Variant To Data(error in=w305, type=w306, Variant=w301) -> (data=w304:u16, error out=w303:errorcluster)
            n91 = property on="step.size.z 2" class="Ring (strict)"(error in=w303, "Value"=w304) -> (error out=w302:errorcluster)  [unwired: 1 in, 1 out]
          }
          frame "channel.no" {
            n92 = Not(x=w313) -> (.not. x?=w312:bool)
            n93 = feedback #1() -> (w321:variant)  [unwired: 1 in]
            n94 = feedback-in #1(w322) -> ()
            n95 = Not Equal?(x=w322, y=w321) -> (x != y?=w315:bool)
            n96 = Or(x=w312, y=w315) -> (x .or. y?=w314:bool)
            n97 = case shown="False" w314 {
              tunnel: w322 -> [_ w353]
              tunnel: w320 -> [w330 w352]
              tunnel: [w331 w351] -> w319
              tunnel: w318 -> [_ w350]
              tunnel: [w330 w349] -> w317
              tunnel: w311 -> [w331 _]
              frame False {
              }
              frame True {
                w339 = refnum<vi> refnum  # Generic
                # "Enable 'Overlay Control' only when there is valid \"current data\""
                # "Validate Image when new data\nis written in the main GUI"
                n98 = Unbundle By Name(w350) -> ("Current Image"=w342:refnum<vi>, "Overlay"=w341:refnum<vi>)
                n99 = Variant To Data(type=0, Variant=w353) -> (data=w338:i32)  [unwired: 1 in, 1 out]
                n100 = To More Generic Class(target class=w339, reference=w342) -> (generic class reference=w343:refnum<vi>)
                n101 = Build Array(w341) -> (w340:refnum<vi>[])
                n102 = call "ImageControl.vi"("Error In"=w352, "Channel No"=w338, "Image Refnum (Generic)"=w343) -> ("Error Out"=w344:errorcluster, "Current Image"=w351:T7)  [unwired: 7 in]
                n103 = case shown="0, Default" w338 {
                  tunnel: [MAIN_Image_panel_tab_Control_type_def."Channel 1" ("Tab IN") MAIN_Image_panel_tab_Control_type_def."Channel 1" ("Tab IN") MAIN_Image_panel_tab_Control_type_def."Channel 2" ("Tab IN") MAIN_Image_panel_tab_Control_type_def."Channel 3" ("Tab IN") MAIN_Image_panel_tab_Control_type_def."Channel 4" ("Tab IN")] -> w336
                  frame 0, Default {
                  }
                  frame 1 {
                  }
                  frame 2 {
                  }
                  frame 3 {
                  }
                  frame 4 {
                  }
                }
                n104 = call "Chnl_2_tab.vi"("Command"=Chnl_2_tab_Commands."TabToChannel", "Error In"=w344, "Tab IN"=w336) -> ("Error Out"=w346:errorcluster, "Channel  OUT"=w345:T5)  [unwired: 6 in, 1 out]
                n105 = property on="Source" class="Enum (strict)"(error in=w346, "Value"=w345) -> (error out=w347:errorcluster)  [unwired: 1 in, 1 out]
                n106 = call "Image Validity FGV.vi"("Image Validity FGV_Commands"=Image_Validity_FGV_Commands."Set validity status", "Error In"=w347, "Validity status IN"=TRUE) -> ("Error Out"=w348:errorcluster)  [unwired: 7 in, 1 out]
                n107 = First Call?() -> (First Call?: T/F=w332:bool)
                n108 = case shown="True" w332 {
                  tunnel: w348 -> [w359 w362]
                  tunnel: [w359 w361] -> w349
                  tunnel: w340 -> [_ w360]
                  frame False {
                  }
                  frame True {
                    n109 = call "UI Control and Indicator properties.vi"("Enable Command"=UI_Control_and_Indicator_properties_Commands."Enable", "Error In"=w362, "Control Refnums"=w360) -> ("Error Out"=w361:errorcluster)  [unwired: 8 in]
                  }
                }
              }
            }
          }
          frame "MAIN.Image.panels.", "MAIN.Image.panels.reso." {
            # "Clear Error  91 if it occurs. Eg. when \nGFG variable for the 'main image panel' of the wrong  type is set - This is triggered by MACRO MODULE"
            n110 = Unbundle By Name(w373) -> ("Source"=w372:refnum<vi>)
            n111 = Variant To Data(error in=w374, type=0, Variant=w379) -> (data=w369:i32, error out=w367:errorcluster)
            n112 = call "Clear Specific Errors.vi"("Error In"=w367, "Error number In"=91) -> ("Error Out"=w366:errorcluster, "Error Cleared?"=w365:bool)  [unwired: 8 in]
            n113 = case shown="True" w365 {
              tunnel: w372 -> [w389 _]
              tunnel: [w388 w397] -> w371
              tunnel: w369 -> [w386 _]
              tunnel: w366 -> [w384 w397]
              frame False {
                n114 = Less?(x=w386, y=4) -> (x < y?=w387:bool)
                n115 = case shown="True" w387 {
                  tunnel: w389 -> [_ w396]
                  tunnel: [w390 w393] -> w388
                  tunnel: w386 -> [_ w392]
                  tunnel: w384 -> [w390 w391]
                  frame False {
                  }
                  frame True {
                    n116 = property class="Enum (strict)"(reference=w396, error in=w391, "Value"=w392) -> (reference out=w394:refnum<vi>, error out=w395:errorcluster)
                    n117 = Close Reference(reference=w394, error in (no error)=w395) -> (error out=w393:errorcluster)
                  }
                }
              }
              frame True {
                # "Error 91 has been cleared.\nWrong 'Image Panels GFG variable' set.\nDO NOTHING!"
              }
            }
          }
          frame "no.of.grid.lines" {
            n118 = Variant To Data(type=0.0 ("no of grid lines 2"), Variant=w401) -> (data=w399:dbl)  [unwired: 1 in, 1 out]
            n119 = local write "no of grid lines 2"(w399) -> ()
            n120 = call "IMAQ Clear Overlay"("Image"=w398) -> ()  [unwired: 9 in, 2 out]
          }
          frame "moveXYZabs" {
            n121 = disable-structure shown="Enabled" {
              disable-tunnel: w420 -> [w434 _]
              disable-tunnel: [w424 w441] -> w419
              disable-tunnel: w417 -> [w425 w441]
              frame Disabled {
                w439 = enum16{"Init", "Set", "Get"}."Set" ("Action")
                # "Set the XYZ positions"
                # "!! ~~~~ Disable this Case on actual H/W~~~~~ !!\n(Used on development environment to simulate an XYZ stage)"
                n122 = Variant To Data(type=T18 {"moveXabs"=0.0, "moveYabs"=0.0, "moveZabs"=0.0} ("output cluster"), Variant=w434) -> (data=w435:T18)  [unwired: 1 in, 1 out]
                n123 = Unbundle By Name(w435) -> ("moveXabs"=w431:dbl, "moveYabs"=w430:dbl, "moveZabs"=w429:dbl)
                n124 = To Variant(anything=w430) -> (Variant=w427:variant)
                n125 = To Variant(anything=w431) -> (Variant=w428:variant)
                n126 = To Variant(anything=w429) -> (Variant=w426:variant)
                n127 = call "GFG_core.vi"("Variable Name in"="posX", "Variant in"=w428, "error in (no error)"=w425, "Action"=w439) -> ("error out"=w432:errorcluster)  [unwired: 9 in, 6 out]
                n128 = call "GFG_core.vi"("Variable Name in"="posY", "Variant in"=w427, "error in (no error)"=w432, "Action"=w439) -> ("error out"=w433:errorcluster)  [unwired: 9 in, 6 out]
                n129 = call "GFG_core.vi"("Variable Name in"="posZ", "Variant in"=w426, "error in (no error)"=w433, "Action"=w439) -> ("error out"=w424:errorcluster)  [unwired: 9 in, 6 out]
              }
              frame Enabled {
              }
            }
          }
          frame "posX", "posY", "posZ" {
            # "Invalidate Image when carriage moves"
            # "Invalidate Image when carriage moves"
            n130 = call "GetCurrentPosition.vi"("Error In"=w454) -> ("Error Out"=w443:errorcluster, "Z"=w457:dbl, "Y"=w456:dbl, "X"=w455:dbl)  [unwired: 7 in]
            n131 = call "Image Validity FGV.vi"("Image Validity FGV_Commands"=Image_Validity_FGV_Commands."Set validity status", "Error In"=w443, "Validity status IN"=FALSE) -> ("Error Out"=w442:errorcluster)  [unwired: 7 in, 1 out]
            n132 = call "GenerateDisplayData.vi"("Index"=w447, "Error In"=w442, "UI Controls Refnum"=w449, "2D Data IN"=w452) -> ("Error Out"=w453:errorcluster, "Plot Data OUT"=w451:cluster{dbl[], dbl[]}[])  [unwired: 4 in, 2 out]
          }
          frame "QUIT" {
            w486 = string[][] [] ("Formatted Table Data")
            w492 = 0.0 ("X")
            # "Reset the button in main UI"
            # "Clear table display"
            n133 = Unbundle By Name(w490) -> ("Big Table"=w484:refnum<vi>, "Notes Table"=w487:refnum<vi>, "Hide"=w479:refnum<vi>)
            n134 = Build Array(w484, w487) -> (w483:refnum<vi>[])
            n135 = call "FormatTableStyle.vi"("Format Command"=FormatTableStyle_Commands."Uncolour Row", "Error In"=w489, "Row Index"=w491, "Table reference Array"=w483) -> ("Error Out"=w488:errorcluster)  [unwired: 7 in]
            n136 = for {
              tunnel: w486 -> [w515]
              shift-right: [w514] -> w476
              shift-left: w488 -> [w518]
              tunnel: w483 -> [w513] mode=indexing
              n137 = property class="Tbl (strict)"(reference=w513, error in=w518, "Value"=w515) -> (reference out=w516:refnum<vi>, error out=w517:errorcluster)
              n138 = Close Reference(reference=w516, error in (no error)=w517) -> (error out=w514:errorcluster)
            }
            n139 = property class="Bool (strict)"(reference=w479, error in=w476, "Value"=T2 FALSE) -> (reference out=w477:refnum<vi>, error out=w478:errorcluster)
            n140 = Close Reference(reference=w477, error in (no error)=w478) -> (error out=w474:errorcluster)
            n141 = control-ref of="This VI"() -> (w461:refnum<vi>)
            n142 = property class="VI"(reference=w461, error in=w474) -> (error out=w459:errorcluster, "FP.State"=w460:T13)  [unwired: 1 out]
            n143 = call "GFGfpRefGet.vi"("Variable Name in"="PositionSaveButton") -> ("output cluster"=w470:T22)  [unwired: 9 in, 1 out]
            n144 = case shown="\"Hidden\"" w460 {
              tunnel: [w493 w496 w501 w506 w509 w510] -> w473
              tunnel: w461 -> [_ w495 w500 w505 _ _]
              tunnel: w459 -> [w493 w494 w499 w504 w509 w510]
              frame "Invalid", Default {
              }
              frame "Standard" {
                n145 = invoke class="VI" method="FP.Close"(reference=w495, error in=w494) -> (reference out=w497:refnum<vi>, error out=w498:errorcluster)  [unwired: 1 in, 1 out]
                n146 = Close Reference(reference=w497, error in (no error)=w498) -> (error out=w496:errorcluster)
              }
              frame "Minimized" {
                n147 = invoke class="VI" method="FP.Close"(reference=w500, error in=w499) -> (reference out=w502:refnum<vi>, error out=w503:errorcluster)  [unwired: 1 in, 1 out]
                n148 = Close Reference(reference=w502, error in (no error)=w503) -> (error out=w501:errorcluster)
              }
              frame "Maximized" {
                n149 = invoke class="VI" method="FP.Close"(reference=w505, error in=w504) -> (reference out=w507:refnum<vi>, error out=w508:errorcluster)  [unwired: 1 in, 1 out]
                n150 = Close Reference(reference=w507, error in (no error)=w508) -> (error out=w506:errorcluster)
              }
              frame "Closed" {
              }
              frame "Hidden" {
              }
            }
            n151 = Unbundle By Name(w470) -> ("BooleanRef"=w466:refnum<vi>)
            n152 = property class="Bool"(reference=w466, "Value"=FALSE) -> (reference out=w467:refnum<vi>, error out=w468:errorcluster)  [unwired: 1 in]
            n153 = Close Reference(reference=w467, error in (no error)=w468) -> (error out=w462:errorcluster)
            n154 = flat-sequence {
              tunnel: w473 -> [w511]
              tunnel: [w511] -> _
              tunnel: [TRUE] -> w465
              tunnel: [w511] -> w463
              frame #0 {
              }
            }
            n155 = Merge Errors(w463, w462) -> (w464:errorcluster)
          }
        }
      }
      event Panel Close? {
        n156 = event-data() -> ()  [unwired: 1 in, 1 out]
        n157 = control-ref of="This VI"() -> (w533:refnum<vi>)
        n158 = property class="VI"(reference=w533, error in=w521, "FP.State"=T13."Hidden" ("Front Panel Window:State")) -> (reference out=w531:refnum<vi>, error out=w532:errorcluster)
        n159 = Close Reference(reference=w531, error in (no error)=w532) -> (error out=w524:errorcluster)
        n160 = call "GFGfpRefGet.vi"("error in (no error)"=w524, "Variable Name in"="PositionSaveButton") -> ("error out"=w528:errorcluster, "output cluster"=w529:T22)  [unwired: 8 in]
        n161 = Unbundle By Name(w529) -> ("BooleanRef"=w527:refnum<vi>)
        n162 = property class="Bool"(reference=w527, error in=w528, "Value"=FALSE) -> (reference out=w525:refnum<vi>, error out=w526:errorcluster)
        n163 = Close Reference(reference=w525, error in (no error)=w526) -> (error out=w520:errorcluster)
        n164 = event-data("Discard?"=TRUE) -> ()  [unwired: 1 in, 1 out]
      }
      event "Overlay": Value Change {
        # "Enable/Disable the Overlay cluster according to\nthe value"
        n165 = event-data() -> ("NewVal"=w550:bool)  [unwired: 1 in]
        n166 = Unbundle By Name(w549) -> ("Overlay Controls"=w548:refnum<vi>)
        n167 = case shown="False" w550 {
          tunnel: w548 -> [w562 w567]
          tunnel: w547 -> [w563 w568]
          tunnel: [w560 w565] -> w546
          frame True {
            n168 = Build Array(w562) -> (w561:refnum<vi>[])
            n169 = call "UI Control and Indicator properties.vi"("Enable Command"=UI_Control_and_Indicator_properties_Commands."Enable", "Error In"=w563, "Control Refnums"=w561) -> ("Error Out"=w560:errorcluster)  [unwired: 8 in]
          }
          frame False {
            n170 = Build Array(w567) -> (w566:refnum<vi>[])
            n171 = call "UI Control and Indicator properties.vi"("Enable Command"=UI_Control_and_Indicator_properties_Commands."Disable and Grey", "Error In"=w568, "Control Refnums"=w566) -> ("Error Out"=w565:errorcluster)  [unwired: 8 in]
          }
        }
      }
      event Value Change {
        # "Make sure the loop executes, to update the Image whenever there is a change in  any of the Overlay controls"
        n172 = event-data() -> ()  [unwired: 1 in, 1 out]
      }
      event "Hor_Cluster.Load List": Value Change {
        w619 = T12 {"CurrentImage"=refnum, "SavedImage"=refnum}  # Image Input Cluster
        # "Stop listening to GFG events during execution of this case"
        # "Update table and plot display"
        n173 = event-data() -> ()  [unwired: 1 in, 1 out]
        n174 = Bundle By Name(cluster=w619, "CurrentImage"=w618, "SavedImage"=w617) -> (w616:T12)
        n175 = call "Register_Unregister_UserEvents_PSMGUI.vi"("Event Registration Refnum IN"=w596, "Action"=enum16{"Register", "Un-Register"}."Un-Register", "error in (no error)"=w597) -> ("Event Registration Refnum OUT"=w590:refnum<event-registration>, "error out"=w594:errorcluster)  [unwired: 8 in, 3 out]
        n176 = call "PositionSaveFGV.vi"("Image Cluster Input"=w616, "PositionSave Commands"=PositionSaveFGVCommands."LoadList", "Error In"=w594) -> ("Error Out"=w623:errorcluster, "SavedImage out"=w615:T7, "cancelled/failed"=w622:bool, "Position Data Out"=w624:string[][], "Path"=w614:path)  [unwired: 4 in]
        n177 = case shown="False" w622 {
          tunnel: w624 -> [w637 _]
          tunnel: w623 -> [w647 w662]
          tunnel: [w639 w662] -> w604
          tunnel: [w637 w661] -> w608
          tunnel: w599 -> [w631 _]
          tunnel: w621 -> [_ w661]
          tunnel: w620 -> [w627 w660]
          tunnel: [w626 w660] -> w607
          frame False {
            # "No of rows > 0?"
            # "Colour only if there\nare entries"
            # "Enable UI components and \nUpdate table and Graph"
            n178 = Unbundle By Name(w631) -> ("Set POI"=w628:refnum<vi>, "Set New Origin"=w652:refnum<vi>, "Delete Item"=w651:refnum<vi>, "Notes Table"=w641:refnum<vi>, "GO TO"=w650:refnum<vi>, "Big Table"=w629:refnum<vi>, "Table Up-End"=w646:refnum<vi>, "Table Up"=w645:refnum<vi>, "Table Down"=w644:refnum<vi>, "Table Down-End"=w643:refnum<vi>, "Copy Button"=w632:refnum<vi>)
            n179 = Build Array(w628, w652, w651, w641, w650, w629, w646, w645, w644, w643, w632) -> (w648:refnum<vi>[])
            n180 = Build Array(w641, w629) -> (w638:refnum<vi>[])
            n181 = call "UI Control and Indicator properties.vi"("Enable Command"=UI_Control_and_Indicator_properties_Commands."Enable", "Error In"=w647, "Control Refnums"=w648) -> ("Error Out"=w630:errorcluster)  [unwired: 8 in]
            n182 = Array Size(array=w637) -> (size(s)=w636:i32[])
            n183 = Index Array(array=w636, index=0) -> (element=w634:i32)
            n184 = Greater Than 0?(x=w634) -> (x > 0?=w633:bool)
            n185 = call "FormatTableStyle.vi"("Format Command"=FormatTableStyle_Commands."Uncolour Row", "Error In"=w630, "Row Index"=w627, "Table reference Array"=w638) -> ("Error Out"=w640:errorcluster)  [unwired: 7 in]
            n186 = case shown="False" w633 {
              tunnel: w640 -> [w654 w659]
              tunnel: [w654 w657] -> w639
              tunnel: w638 -> [_ w656]
              tunnel: [-1 ("Row") w655] -> w626
              frame False {
              }
              frame True {
                w655 = 0 ("Row")
                n187 = call "FormatTableStyle.vi"("Format Command"=FormatTableStyle_Commands."Colour Row", "Error In"=w659, "Row Index"=w655, "Table reference Array"=w656) -> ("Error Out"=w657:errorcluster)  [unwired: 7 in]
              }
            }
          }
          frame True {
            # "Action cancelled by user\n- Do nothing"
          }
        }
        n188 = call "GenerateDisplayData.vi"("Index"=w607, "Error In"=w604, "UI Controls Refnum"=w599, "2D Data IN"=w608) -> ("Error Out"=w600:errorcluster, "Notes"=w601:string[][], "Big Table"=w611:string[][], "Plot Data OUT"=w606:cluster{dbl[], dbl[]}[])  [unwired: 4 in]
        n189 = Unbundle By Name(w599) -> ("Big Table"=w605:refnum<vi>, "Notes Table"=w602:refnum<vi>)
        n190 = property class="Tbl (strict)"(reference=w605, error in=w600, "Value"=w611) -> (reference out=w612:refnum<vi>, error out=w613:errorcluster)
        n191 = Close Reference(reference=w612, error in (no error)=w613) -> (error out=w603:errorcluster)
        n192 = property class="Tbl (strict)"(reference=w602, error in=w603, "Value"=w601) -> (reference out=w609:refnum<vi>, error out=w610:errorcluster)
        n193 = Close Reference(reference=w609, error in (no error)=w610) -> (error out=w591:errorcluster)
        n194 = call "Register_Unregister_UserEvents_PSMGUI.vi"("Event Registration Refnum IN"=w590, "Action"=enum16{"Register", "Un-Register"}."Register", "Pos X IN"=w588, "Pos Y IN"=w587, "Pos Z IN"=w586, "error in (no error)"=w591) -> ("Event Registration Refnum OUT"=w589:refnum<event-registration>, "Pos X OUT"=w585:dbl, "Pos Y OUT"=w584:dbl, "Pos Z  OUT"=w583:dbl, "error out"=w592:errorcluster)  [unwired: 5 in]
      }
      event "Hor_Cluster.New List": Value Change {
        n195 = event-data() -> ()  [unwired: 1 in, 1 out]
        n196 = Bundle By Name(cluster=T12 {"CurrentImage"=refnum, "SavedImage"=refnum} ("Image Cluster Input"), "CurrentImage"=w689, "SavedImage"=w690) -> (w688:T12)
        n197 = call "Register_Unregister_UserEvents_PSMGUI.vi"("Event Registration Refnum IN"=w676, "Action"=enum16{"Register", "Un-Register"}."Un-Register", "error in (no error)"=w677) -> ("Event Registration Refnum OUT"=w671:refnum<event-registration>, "error out"=w675:errorcluster)  [unwired: 8 in, 3 out]
        n198 = call "PositionSaveFGV.vi"("Image Cluster Input"=w688, "PositionSave Commands"=PositionSaveFGVCommands."NewList", "Error In"=w675) -> ("Error Out"=w694:errorcluster, "SavedImage out"=w687:T7, "cancelled/failed"=w693:bool, "Position Data Out"=w695:string[][], "Path"=w685:path)  [unwired: 4 in]
        n199 = case shown="False" w693 {
          tunnel: w695 -> [w707 _]
          tunnel: w694 -> [w719 w730]
          tunnel: [w704 w730] -> w684
          tunnel: [w707 w729] -> w683
          tunnel: w680 -> [w698 _]
          tunnel: w692 -> [_ w729]
          tunnel: w691 -> [w712 w728]
          tunnel: [0 ("Row") w728] -> w681
          frame False {
            # "Enable UI components and \nUpdate table and Graph"
            n200 = Unbundle By Name(w698) -> ("Set New Origin"=w699:refnum<vi>, "Notes Table"=w700:refnum<vi>, "Big Table"=w711:refnum<vi>, "Table Up-End"=w718:refnum<vi>, "Table Up"=w717:refnum<vi>, "Table Down"=w716:refnum<vi>, "Table Down-End"=w715:refnum<vi>, "Copy Button"=w701:refnum<vi>)  [unwired: 1 out]
            n201 = Build Array(w700, w711) -> (w708:refnum<vi>[])
            n202 = Build Array(w699, w700, w711, w718, w717, w716, w715, w701) -> (w720:refnum<vi>[])
            n203 = call "UI Control and Indicator properties.vi"("Enable Command"=UI_Control_and_Indicator_properties_Commands."Enable", "Error In"=w719, "Control Refnums"=w720) -> ("Error Out"=w697:errorcluster)  [unwired: 8 in]
            n204 = call "FormatTableStyle.vi"("Format Command"=FormatTableStyle_Commands."Uncolour Row", "Error In"=w697, "Row Index"=w712, "Table reference Array"=w708) -> ("Error Out"=w710:errorcluster)  [unwired: 7 in]
            n205 = for {
              tunnel: string[][] [] ("Value") -> [w726]
              shift-right: [w723] -> w703
              shift-left: w710 -> [w727]
              tunnel: w708 -> [w722] mode=indexing
              n206 = property class="Tbl (strict)"(reference=w722, error in=w727, "Value"=w726) -> (reference out=w724:refnum<vi>, error out=w725:errorcluster)
              n207 = Close Reference(reference=w724, error in (no error)=w725) -> (error out=w723:errorcluster)
            }
            n208 = property class="Bool"(reference=w699, error in=w703, "Blinking"=TRUE) -> (reference out=w705:refnum<vi>, error out=w706:errorcluster)
            n209 = Close Reference(reference=w705, error in (no error)=w706) -> (error out=w704:errorcluster)
          }
          frame True {
            # "Action cancelled by user\n- Do nothing"
          }
        }
        n210 = call "GenerateDisplayData.vi"("Index"=w681, "Error In"=w684, "UI Controls Refnum"=w680, "2D Data IN"=w683) -> ("Error Out"=w673:errorcluster, "Plot Data OUT"=w682:cluster{dbl[], dbl[]}[])  [unwired: 4 in, 2 out]
        n211 = call "Register_Unregister_UserEvents_PSMGUI.vi"("Event Registration Refnum IN"=w671, "Action"=enum16{"Register", "Un-Register"}."Register", "Pos X IN"=w669, "Pos Y IN"=w668, "Pos Z IN"=w667, "error in (no error)"=w673) -> ("Event Registration Refnum OUT"=w670:refnum<event-registration>, "Pos X OUT"=w666:dbl, "Pos Y OUT"=w665:dbl, "Pos Z  OUT"=w664:dbl, "error out"=w672:errorcluster)  [unwired: 5 in]
      }
      event "Hor_Cluster.Set new Origin": Value Change {
        w764 = T12 {"CurrentImage"=refnum, "SavedImage"=refnum}  # Image Input Cluster
        # "Is there any data in the\nlist?"
        # "If the image is not up-to-date donot set POI!"
        n212 = event-data() -> ()  [unwired: 1 in, 1 out]
        n213 = Array Size(array=w756) -> (size(s)=w755:i32[])
        n214 = Bundle By Name(cluster=w764, "CurrentImage"=w762, "SavedImage"=w763) -> (w761:T12)
        n215 = call "Register_Unregister_UserEvents_PSMGUI.vi"("Event Registration Refnum IN"=w743, "Action"=enum16{"Register", "Un-Register"}."Un-Register", "error in (no error)"=w745) -> ("Event Registration Refnum OUT"=w740:refnum<event-registration>, "error out"=w744:errorcluster)  [unwired: 8 in, 3 out]
        n216 = Index Array(array=w755, index=0) -> (element=w753:i32)
        n217 = call "Image Validity FGV.vi"("Image Validity FGV_Commands"=Image_Validity_FGV_Commands."Get Validity status", "Error In"=w744) -> ("Error Out"=w758:errorcluster, "Validity status OUT"=w757:bool)  [unwired: 8 in]
        n218 = Greater Than 0?(x=w753) -> (x > 0?=w752:bool)
        n219 = case shown="True" w757 {
          tunnel: w771 -> [w775 w789]
          tunnel: w770 -> [w774 w788]
          tunnel: w760 -> [w773 w787]
          tunnel: w758 -> [w780 w785]
          tunnel: [w781 w800] -> w769
          tunnel: w751 -> [_ w799]
          tunnel: [w780 w798] -> w742
          tunnel: w756 -> [w781 w797]
          tunnel: w768 -> [w779 w795]
          tunnel: [w779 w794] -> w767
          tunnel: w766 -> [w776 w793]
          tunnel: [w776 w792] -> w765
          tunnel: w761 -> [w778 w791]
          tunnel: [w777 w790] -> w748
          tunnel: [w775 w789] -> w737
          tunnel: [w774 w788] -> w736
          tunnel: [w773 w787] -> w735
          tunnel: w752 -> [_ w786]
          tunnel: [w772 w784] -> w750
          tunnel: w749 -> [w772 w783]
          frame False {
            n220 = Unbundle By Name(w778) -> ("SavedImage"=w777:T7)
            n221 = call "Dialog_ImageNotUptodate_Error.vi"() -> ()  [unwired: 12 in]
          }
          frame True {
            w802 = T20 {"X"=0.0, "Y"=0.0, "Z"=0.0, "Base Path"=path ""}  # Position Data In
            # "Takes the current XYZ position and updates the table data on user confirmation"
            n222 = case shown="True" w786 {
              selector: w786 -> [w803 w806]
              tunnel: [TRUE ("T button?") w805] -> w796
              tunnel: [w803 w806] -> w782
              frame False {
              }
              frame True {
                n223 = call "Dialog_SetNewOrigin.vi"() -> ("OK?"=w805:bool)  [unwired: 11 in]
              }
            }
            n224 = Bundle By Name(cluster=w802, "X"=w789, "Y"=w788, "Z"=w787) -> (w801:T20)
            n225 = case shown="True" w796 {
              tunnel: w785 -> [w812 w853]
              tunnel: w801 -> [_ w852]
              tunnel: [w813 w851] -> w800
              tunnel: w799 -> [_ w816]
              tunnel: [w812 w821] -> w798
              tunnel: w797 -> [w813 _]
              tunnel: w795 -> [w811 w815]
              tunnel: [w811 w840] -> w794
              tunnel: w793 -> [w810 _]
              tunnel: [w810 w831] -> w792
              tunnel: w791 -> [w809 w830]
              tunnel: [w808 w829] -> w790
              tunnel: [w807 w818] -> w784
              tunnel: w783 -> [w807 _]
              tunnel: w782 -> [_ w817]
              frame False {
                n226 = Unbundle By Name(w809) -> ("SavedImage"=w808:T7)
              }
              frame True {
                w840 = 0 ("Row Index")
                # "If this is a new data file,\nenable the 'Go To' and 'Delete buttons'"
                n227 = call "PositionSaveFGV.vi"("Image Cluster Input"=w830, "PositionSave Commands"=PositionSaveFGVCommands."SetNewOrigin", "Error In"=w853, "Position Data In"=w852) -> ("Error Out"=w832:errorcluster, "SavedImage out"=w829:T7, "Position Data Out"=w851:string[][], "Path"=w818:path)  [unwired: 3 in, 1 out]
                n228 = Unbundle By Name(w816) -> ("Big Table"=w849:refnum<vi>, "Notes Table"=w836:refnum<vi>, "Set New Origin"=w827:refnum<vi>, "Set POI"=w823:refnum<vi>)
                n229 = case shown="False" w817 {
                  tunnel: w816 -> [w859 _]
                  frame False {
                    n230 = Unbundle By Name(w859) -> ("GO TO"=w857:refnum<vi>, "Delete Item"=w856:refnum<vi>)
                    n231 = Build Array(w857, w856) -> (w855:refnum<vi>[])
                    n232 = call "UI Control and Indicator properties.vi"("Enable Command"=UI_Control_and_Indicator_properties_Commands."Enable", "Control Refnums"=w855) -> ()  [unwired: 9 in, 1 out]
                  }
                  frame True {
                  }
                }
                n233 = call "GenerateDisplayData.vi"("Index"=0, "Error In"=w832, "UI Controls Refnum"=w816, "2D Data IN"=w851) -> ("Error Out"=w850:errorcluster, "Notes"=w833:string[][], "Big Table"=w834:string[][], "Plot Data OUT"=w831:cluster{dbl[], dbl[]}[])  [unwired: 4 in]
                n234 = property class="Tbl (strict)"(reference=w849, error in=w850, "Value"=w834) -> (reference out=w847:refnum<vi>, error out=w848:errorcluster)
                n235 = Build Array(w849, w836) -> (w842:refnum<vi>[])
                n236 = Build Array(w823) -> (w820:refnum<vi>[])
                n237 = Close Reference(reference=w847, error in (no error)=w848) -> (error out=w839:errorcluster)
                n238 = property class="Tbl (strict)"(reference=w836, error in=w839, "Value"=w833) -> (reference out=w837:refnum<vi>, error out=w838:errorcluster)
                n239 = Close Reference(reference=w837, error in (no error)=w838) -> (error out=w835:errorcluster)
                n240 = call "FormatTableStyle.vi"("Format Command"=FormatTableStyle_Commands."Uncolour Row", "Error In"=w835, "Row Index"=w815, "Table reference Array"=w842) -> ("Error Out"=w843:errorcluster)  [unwired: 7 in]
                n241 = call "FormatTableStyle.vi"("Format Command"=FormatTableStyle_Commands."Colour Row", "Error In"=w843, "Row Index"=w840, "Table reference Array"=w842) -> ("Error Out"=w841:errorcluster)  [unwired: 7 in]
                n242 = call "FormatTableStyle.vi"("Format Command"=FormatTableStyle_Commands."UpdateVisibleRows", "Error In"=w841, "Row Index"=w840, "Table reference Array"=w842) -> ("Error Out"=w828:errorcluster)  [unwired: 7 in]
                n243 = property class="Bool"(reference=w827, error in=w828, "Blinking"=FALSE) -> (reference out=w824:refnum<vi>, error out=w825:errorcluster)
                n244 = Close Reference(reference=w824, error in (no error)=w825) -> (error out=w822:errorcluster)
                n245 = call "UI Control and Indicator properties.vi"("Enable Command"=UI_Control_and_Indicator_properties_Commands."Enable", "Error In"=w822, "Control Refnums"=w820) -> ("Error Out"=w821:errorcluster)  [unwired: 8 in]
              }
            }
          }
        }
        n246 = call "Register_Unregister_UserEvents_PSMGUI.vi"("Event Registration Refnum IN"=w740, "Action"=enum16{"Register", "Un-Register"}."Register", "Pos X IN"=w737, "Pos Y IN"=w736, "Pos Z IN"=w735, "error in (no error)"=w742) -> ("Event Registration Refnum OUT"=w738:refnum<event-registration>, "Pos X OUT"=w734:dbl, "Pos Y OUT"=w733:dbl, "Pos Z  OUT"=w732:dbl, "error out"=w739:errorcluster)  [unwired: 5 in]
      }
      event "Copy Button": Value Change {
        w882 = T12 {"CurrentImage"=refnum, "SavedImage"=refnum}  # Image Input Cluster
        # "Makes a copy of the csv file to user specified destination. For implementation details check the PositionSaveFGV."
        n247 = event-data() -> ()  [unwired: 1 in, 1 out]
        n248 = call "Register_Unregister_UserEvents_PSMGUI.vi"("Event Registration Refnum IN"=w869, "Action"=enum16{"Register", "Un-Register"}."Un-Register", "error in (no error)"=w871) -> ("Event Registration Refnum OUT"=w868:refnum<event-registration>, "error out"=w870:errorcluster)  [unwired: 8 in, 3 out]
        n249 = Bundle By Name(cluster=w882, "CurrentImage"=w881, "SavedImage"=w880) -> (w879:T12)
        n250 = call "PositionSaveFGV.vi"("Image Cluster Input"=w879, "PositionSave Commands"=PositionSaveFGVCommands."CopyList", "Error In"=w870) -> ("Error Out"=w891:errorcluster, "SavedImage out"=w878:T7, "cancelled/failed"=w887:bool, "Position Data Out"=w892:string[][], "Path"=w877:path)  [unwired: 4 in]
        n251 = case shown="False" w887 {
          tunnel: w892 -> [w905 _]
          tunnel: w891 -> [w921 w937]
          tunnel: [w908 w937] -> w873
          tunnel: [w905 w936] -> w890
          tunnel: [w900 w938] -> w889
          tunnel: w888 -> [_ w938]
          tunnel: w886 -> [w895 _]
          tunnel: w885 -> [_ w936]
          tunnel: w884 -> [w894 w935]
          tunnel: [w906 w935] -> w883
          frame False {
            w906 = 0 ("Row")
            # "No of rows > 0?"
            # "Colour only if there\nare entries"
            # "Enable UI components and \nUpdate table and Graph"
            n252 = Unbundle By Name(w895) -> ("Set POI"=w897:refnum<vi>, "Set New Origin"=w928:refnum<vi>, "Delete Item"=w927:refnum<vi>, "Notes Table"=w912:refnum<vi>, "GO TO"=w926:refnum<vi>, "Big Table"=w911:refnum<vi>, "Table Up-End"=w920:refnum<vi>, "Table Up"=w919:refnum<vi>, "Table Down"=w918:refnum<vi>, "Table Down-End"=w917:refnum<vi>, "Copy Button"=w896:refnum<vi>)
            n253 = Build Array(w897, w928, w927, w912, w926, w911, w920, w919, w918, w917, w896) -> (w924:refnum<vi>[])
            n254 = call "UI Control and Indicator properties.vi"("Enable Command"=UI_Control_and_Indicator_properties_Commands."Enable", "Error In"=w921, "Control Refnums"=w924) -> ("Error Out"=w923:errorcluster)  [unwired: 8 in]
            n255 = call "GenerateDisplayData.vi"("Index"=w894, "Error In"=w923, "UI Controls Refnum"=w895, "2D Data IN"=w905) -> ("Error Out"=w922:errorcluster, "Notes"=w898:string[][], "Big Table"=w899:string[][], "Plot Data OUT"=w900:cluster{dbl[], dbl[]}[])  [unwired: 4 in]
            n256 = property on="Notes_Table" class="Tbl (strict)"(error in=w922, "Value"=w898) -> (error out=w916:errorcluster)  [unwired: 1 in, 1 out]
            n257 = Build Array(w912, w911) -> (w907:refnum<vi>[])
            n258 = property class="Tbl (strict)"(reference=w911, error in=w916, "Value"=w899) -> (reference out=w914:refnum<vi>, error out=w915:errorcluster)
            n259 = Array Size(array=w905) -> (size(s)=w904:i32[])
            n260 = Close Reference(reference=w914, error in (no error)=w915) -> (error out=w910:errorcluster)
            n261 = Index Array(array=w904, index=0) -> (element=w902:i32)
            n262 = Greater Than 0?(x=w902) -> (x > 0?=w901:bool)
            n263 = call "FormatTableStyle.vi"("Format Command"=FormatTableStyle_Commands."Uncolour Row", "Error In"=w910, "Row Index"=w894, "Table reference Array"=w907) -> ("Error Out"=w909:errorcluster)  [unwired: 7 in]
            n264 = case shown="True" w901 {
              tunnel: w909 -> [w929 w934]
              tunnel: [w929 w932] -> w908
              tunnel: w907 -> [_ w931]
              tunnel: w906 -> [_ w930]
              frame False {
              }
              frame True {
                n265 = call "FormatTableStyle.vi"("Format Command"=FormatTableStyle_Commands."Colour Row", "Error In"=w934, "Row Index"=w930, "Table reference Array"=w931) -> ("Error Out"=w932:errorcluster)  [unwired: 7 in]
              }
            }
          }
          frame True {
            # "Action cancelled by user\n- Do nothing"
          }
        }
        n266 = call "Register_Unregister_UserEvents_PSMGUI.vi"("Event Registration Refnum IN"=w868, "Action"=enum16{"Register", "Un-Register"}."Register", "Pos X IN"=w866, "Pos Y IN"=w865, "Pos Z IN"=w864, "error in (no error)"=w873) -> ("Event Registration Refnum OUT"=w867:refnum<event-registration>, "Pos X OUT"=w863:dbl, "Pos Y OUT"=w862:dbl, "Pos Z  OUT"=w861:dbl, "error out"=w872:errorcluster)  [unwired: 5 in]
      }
      event "Vert_Cluster.SET POI": Value Change {
        w975 = T12 {"CurrentImage"=refnum, "SavedImage"=refnum}  # Image Input Cluster
        # "Update plot and table"
        # "If the image is not up-to-date\ndonot set POI!"
        n267 = event-data() -> ()  [unwired: 1 in, 1 out]
        n268 = call "Register_Unregister_UserEvents_PSMGUI.vi"("Event Registration Refnum IN"=w951, "Action"=enum16{"Register", "Un-Register"}."Un-Register", "error in (no error)"=w953) -> ("Event Registration Refnum OUT"=w947:refnum<event-registration>, "error out"=w952:errorcluster)  [unwired: 8 in, 3 out]
        n269 = call "Image Validity FGV.vi"("Image Validity FGV_Commands"=Image_Validity_FGV_Commands."Get Validity status", "Error In"=w952) -> ("Error Out"=w970:errorcluster, "Validity status OUT"=w968:bool)  [unwired: 8 in]
        n270 = Bundle By Name(cluster=w975, "CurrentImage"=w974, "SavedImage"=w973) -> (w972:T12)
        n271 = case shown="True" w968 {
          tunnel: w970 -> [w980 w998]
          tunnel: w957 -> [_ w986]
          tunnel: w977 -> [w981 w997]
          tunnel: [w979 w996] -> w959
          tunnel: [w980 w995] -> w961
          tunnel: [w981 w994] -> w958
          tunnel: [w982 w993] -> w976
          tunnel: w972 -> [w983 w992]
          tunnel: w971 -> [w979 w984]
          tunnel: [w978 w991] -> w967
          tunnel: w966 -> [w978 w985]
          frame False {
            n272 = Unbundle By Name(w983) -> ("SavedImage"=w982:T7)
            n273 = call "Dialog_ImageNotUptodate_Error.vi"() -> ()  [unwired: 12 in]
          }
          frame True {
            # "Are there any saved\ndata points?"
            n274 = Array Size(array=w984) -> (size(s)=w990:i32[])
            n275 = Index Array(array=w990, index=0) -> (element=w988:i32)
            n276 = Greater Than 0?(x=w988) -> (x > 0?=w987:bool)
            n277 = case shown="True" w987 {
              tunnel: w998 -> [w1002 w1029]
              tunnel: w986 -> [_ w1007]
              tunnel: w997 -> [w1001 w1006]
              tunnel: [w999 w1019] -> w996
              tunnel: [w1002 w1015] -> w995
              tunnel: [w1001 w1014] -> w994
              tunnel: [w1003 w1013] -> w993
              tunnel: w992 -> [w1004 w1012]
              tunnel: [w1000 w1008] -> w991
              tunnel: w985 -> [w1000 _]
              tunnel: w984 -> [w999 _]
              frame False {
                n278 = Unbundle By Name(w1004) -> ("SavedImage"=w1003:T7)
                n279 = call "Dialog_NoOrigin_Error.vi"() -> ()  [unwired: 12 in]
              }
              frame True {
                # "If there is atleast one row, add changes to the UI and update index acordingly"
                n280 = call "GetCurrentPosition.vi"("Error In"=w1029) -> ("Error Out"=w1023:errorcluster, "Z"=w1024:dbl, "Y"=w1025:dbl, "X"=w1026:dbl)  [unwired: 7 in]
                n281 = Unbundle By Name(w1007) -> ("Big Table"=w1021:refnum<vi>, "Notes Table"=w1020:refnum<vi>, "Set New Origin"=w1009:refnum<vi>)
                n282 = Bundle By Name(cluster=T20 {"X"=0.0, "Y"=0.0, "Z"=0.0, "Base Path"=path ""} ("Position Data In"), "X"=w1026, "Y"=w1025, "Z"=w1024) -> (w1022:T20)
                n283 = call "PositionSaveFGV.vi"("Image Cluster Input"=w1012, "PositionSave Commands"=PositionSaveFGVCommands."SetPosition", "Error In"=w1023, "Position Data In"=w1022) -> ("Error Out"=w1005:errorcluster, "SavedImage out"=w1013:T7, "Position Data Out"=w1019:string[][], "Path"=w1008:path)  [unwired: 3 in, 1 out]
                n284 = Build Array(w1021, w1020) -> (w1016:refnum<vi>[])
                n285 = Array Size(array=w1019) -> (size(s)=w1018:i32[])
                n286 = Index Array(array=w1018, index=0) -> (element=w1011:i32)
                n287 = Greater Than 0?(x=w1011) -> (x > 0?=w1010:bool)
                n288 = case shown="True" w1010 {
                  tunnel: w1006 -> [_ w1046]
                  tunnel: w1005 -> [w1031 w1044]
                  tunnel: w1016 -> [_ w1040]
                  tunnel: [w1031 w1037] -> w1015
                  tunnel: [w1030 w1039] -> w1014
                  tunnel: w1011 -> [w1030 w1038]
                  tunnel: w1009 -> [_ w1034]
                  frame False {
                  }
                  frame True {
                    n289 = Decrement(x=w1038) -> (x-1=w1039:i32)
                    n290 = call "FormatTableStyle.vi"("Format Command"=FormatTableStyle_Commands."Uncolour Row", "Error In"=w1044, "Row Index"=w1046, "Table reference Array"=w1040) -> ("Error Out"=w1041:errorcluster)  [unwired: 7 in]
                    n291 = call "FormatTableStyle.vi"("Format Command"=FormatTableStyle_Commands."Colour Row", "Error In"=w1041, "Row Index"=w1039, "Table reference Array"=w1040) -> ("Error Out"=w1042:errorcluster)  [unwired: 7 in]
                    n292 = call "FormatTableStyle.vi"("Format Command"=FormatTableStyle_Commands."UpdateVisibleRows", "Error In"=w1042, "Row Index"=w1039, "Table reference Array"=w1040) -> ("Error Out"=w1033:errorcluster)  [unwired: 7 in]
                    n293 = property class="Bool"(reference=w1034, error in=w1033, "Blinking"=FALSE) -> (reference out=w1035:refnum<vi>, error out=w1036:errorcluster)
                    n294 = Close Reference(reference=w1035, error in (no error)=w1036) -> (error out=w1037:errorcluster)
                  }
                }
              }
            }
          }
        }
        n295 = Unbundle By Name(w957) -> ("Big Table"=w960:refnum<vi>)
        n296 = call "GenerateDisplayData.vi"("Index"=w958, "Error In"=w961, "UI Controls Refnum"=w957, "2D Data IN"=w959) -> ("Error Out"=w965:errorcluster, "Big Table"=w962:string[][], "Plot Data OUT"=w956:cluster{dbl[], dbl[]}[])  [unwired: 4 in, 1 out]
        n297 = property class="Tbl (strict)"(reference=w960, error in=w965, "Value"=w962) -> (reference out=w963:refnum<vi>, error out=w964:errorcluster)
        n298 = Close Reference(reference=w963, error in (no error)=w964) -> (error out=w949:errorcluster)
        n299 = call "Register_Unregister_UserEvents_PSMGUI.vi"("Event Registration Refnum IN"=w947, "Action"=enum16{"Register", "Un-Register"}."Register", "Pos X IN"=w945, "Pos Y IN"=w944, "Pos Z IN"=w943, "error in (no error)"=w949) -> ("Event Registration Refnum OUT"=w946:refnum<event-registration>, "Pos X OUT"=w942:dbl, "Pos Y OUT"=w941:dbl, "Pos Z  OUT"=w940:dbl, "error out"=w948:errorcluster)  [unwired: 5 in]
      }
      event "Vert_Cluster.Delete item": Value Change {
        # "Is there any saved positions? (Other than origin)"
        n300 = event-data() -> ()  [unwired: 1 in, 1 out]
        n301 = call "Register_Unregister_UserEvents_PSMGUI.vi"("Event Registration Refnum IN"=w1060, "Action"=enum16{"Register", "Un-Register"}."Un-Register", "error in (no error)"=w1062) -> ("Event Registration Refnum OUT"=w1055:refnum<event-registration>, "error out"=w1061:errorcluster)  [unwired: 8 in, 3 out]
        n302 = Bundle By Name(cluster=T12 {"CurrentImage"=refnum, "SavedImage"=refnum} ("Image Input Cluster"), "SavedImage"=w1071, "CurrentImage"=w1070) -> (w1069:T12)
        n303 = Greater Than 0?(x=w1073) -> (x > 0?=w1067:bool)
        n304 = case shown="True" w1067 {
          selector: w1067 -> [w1080 _]
          tunnel: w1073 -> [w1085 w1100]
          tunnel: w1079 -> [w1086 w1101]
          tunnel: w1061 -> [w1087 w1099]
          tunnel: [w1086 w1098] -> w1078
          tunnel: [w1085 w1097] -> w1077
          tunnel: w1076 -> [_ w1096]
          tunnel: [w1087 w1095] -> w1058
          tunnel: [w1084 w1094] -> w1075
          tunnel: w1074 -> [w1084 w1093]
          tunnel: w1069 -> [w1083 w1092]
          tunnel: [w1082 w1091] -> w1068
          tunnel: [w1081 w1090] -> w1066
          tunnel: w1065 -> [w1081 w1089]
          frame False {
            n305 = Unbundle By Name(w1083) -> ("SavedImage"=w1082:T7)
            n306 = case shown="False" w1080 {
              frame False {
                n307 = call "Dialog_DeleteOrigin_Error.vi"() -> ()  [unwired: 12 in]
              }
              frame True {
              }
            }
          }
          frame True {
            n308 = call "Dialog_DeleteConfirm.vi"() -> ("OK?"=w1088:bool)  [unwired: 11 in]
            n309 = case shown="True" w1088 {
              tunnel: w1101 -> [w1108 w1123]
              tunnel: w1100 -> [w1107 w1111]
              tunnel: w1099 -> [w1106 w1122]
              tunnel: [w1108 w1120] -> w1098
              tunnel: [w1107 w1110] -> w1097
              tunnel: w1096 -> [_ w1121]
              tunnel: [w1106 w1119] -> w1095
              tunnel: [w1105 w1117] -> w1094
              tunnel: w1093 -> [w1105 w1116]
              tunnel: w1092 -> [w1104 w1114]
              tunnel: [w1103 w1113] -> w1091
              tunnel: [w1102 w1109] -> w1090
              tunnel: w1089 -> [w1102 _]
              frame False {
                n310 = Unbundle By Name(w1104) -> ("SavedImage"=w1103:T7)
              }
              frame True {
                n311 = call "PositionSaveFGV.vi"("Image Cluster Input"=w1114, "PositionSave Commands"=PositionSaveFGVCommands."DeleteSelected", "Error In"=w1122, "CompleteTableString"=w1123, "Table Index"=w1111) -> ("Error Out"=w1118:errorcluster, "SavedImage out"=w1113:T7, "cancelled/failed"=w1115:bool, "Position Data Out"=w1120:string[][], "Path"=w1109:path)  [unwired: 2 in]
                n312 = Decrement(x=w1111) -> (x-1=w1112:i32)
                n313 = case shown="False" w1115 {
                  tunnel: w1121 -> [w1126 _]
                  tunnel: w1120 -> [w1139 _]
                  tunnel: [w1132 w1150] -> w1119
                  tunnel: w1118 -> [w1129 w1150]
                  tunnel: [w1128 w1151] -> w1117
                  tunnel: w1116 -> [_ w1151]
                  tunnel: w1112 -> [w1125 _]
                  tunnel: w1111 -> [w1127 w1149]
                  tunnel: [w1125 w1149] -> w1110
                  frame False {
                    n314 = Unbundle By Name(w1126) -> ("Big Table"=w1138:refnum<vi>, "Notes Table"=w1136:refnum<vi>)
                    n315 = call "GenerateDisplayData.vi"("Index"=w1125, "Error In"=w1129, "UI Controls Refnum"=w1126, "2D Data IN"=w1139) -> ("Error Out"=w1137:errorcluster, "Notes"=w1131:string[][], "Big Table"=w1130:string[][], "Plot Data OUT"=w1128:cluster{dbl[], dbl[]}[])  [unwired: 4 in]
                    n316 = property class="Tbl (strict)"(reference=w1138, error in=w1137, "Value"=w1130) -> (reference out=w1143:refnum<vi>, error out=w1142:errorcluster)
                    n317 = Close Reference(reference=w1143, error in (no error)=w1142) -> (error out=w1141:errorcluster)
                    n318 = property class="Tbl (strict)"(reference=w1136, error in=w1141, "Value"=w1131) -> (reference out=w1144:refnum<vi>, error out=w1145:errorcluster)
                    n319 = Build Array(w1138, w1136) -> (w1133:refnum<vi>[])
                    n320 = Close Reference(reference=w1144, error in (no error)=w1145) -> (error out=w1140:errorcluster)
                    n321 = call "FormatTableStyle.vi"("Format Command"=FormatTableStyle_Commands."Uncolour Row", "Error In"=w1140, "Row Index"=w1127, "Table reference Array"=w1133) -> ("Error Out"=w1147:errorcluster)  [unwired: 7 in]
                    n322 = call "FormatTableStyle.vi"("Format Command"=FormatTableStyle_Commands."Colour Row", "Error In"=w1147, "Row Index"=w1125, "Table reference Array"=w1133) -> ("Error Out"=w1135:errorcluster)  [unwired: 7 in]
                    n323 = call "FormatTableStyle.vi"("Format Command"=FormatTableStyle_Commands."UpdateVisibleRows", "Error In"=w1135, "Row Index"=w1125, "Table reference Array"=w1133) -> ("Error Out"=w1132:errorcluster)  [unwired: 7 in]
                  }
                  frame True {
                  }
                }
              }
            }
          }
        }
        n324 = call "Register_Unregister_UserEvents_PSMGUI.vi"("Event Registration Refnum IN"=w1055, "Action"=enum16{"Register", "Un-Register"}."Register", "Pos X IN"=w1054, "Pos Y IN"=w1053, "Pos Z IN"=w1052, "error in (no error)"=w1058) -> ("Event Registration Refnum OUT"=w1056:refnum<event-registration>, "Pos X OUT"=w1051:dbl, "Pos Y OUT"=w1050:dbl, "Pos Z  OUT"=w1049:dbl, "error out"=w1057:errorcluster)  [unwired: 5 in]
      }
      event "Big_Table": Mouse Up {
        w1165 = T12 {"CurrentImage"=refnum, "SavedImage"=refnum}  # Image Input Cluster
        # "Did user click on a row within the data range?"
        n325 = event-data() -> ()  [unwired: 1 in, 1 out]
        n326 = Bundle By Name(cluster=w1165, "SavedImage"=w1164, "CurrentImage"=w1163) -> (w1162:T12)
        n327 = Unbundle By Name(w1154) -> ("Big Table"=w1171:refnum<vi>, "Notes Table"=w1172:refnum<vi>)
        n328 = Array Size(array=w1158) -> (size(s)=w1169:i32[])
        n329 = Index Array(array=w1169, index=0) -> (element=w1168:i32)
        n330 = Decrement(x=w1168) -> (x-1=w1177:i32)
        n331 = property class="Tbl (strict)"(reference=w1171, error in=w1179) -> (reference out=w1174:refnum<vi>, error out=w1175:errorcluster, "Selection Start"=w1178:T23)
        n332 = Build Array(w1171, w1172) -> (w1170:refnum<vi>[])
        n333 = Close Reference(reference=w1174, error in (no error)=w1175) -> (error out=w1173:errorcluster)
        n334 = Unbundle By Name(w1178) -> ("Row"=w1167:i32)
        n335 = Less Or Equal?(x=w1167, y=w1177) -> (x <= y?=w1166:bool)
        n336 = case shown="True" w1166 {
          tunnel: w1167 -> [_ w1189]
          tunnel: w1176 -> [w1187 w1200]
          tunnel: [w1187 w1189] -> w1156
          tunnel: w1173 -> [w1186 w1203]
          tunnel: w1170 -> [_ w1202]
          tunnel: [w1186 w1192] -> w1159
          tunnel: [w1184 w1191] -> w1161
          tunnel: w1158 -> [_ w1190]
          tunnel: w1162 -> [w1185 w1188]
          frame False {
            n337 = Unbundle By Name(w1185) -> ("SavedImage"=w1184:T7)
          }
          frame True {
            # "Update index, and highlight\ntable"
            n338 = call "FormatTableStyle.vi"("Format Command"=FormatTableStyle_Commands."Uncolour Row", "Error In"=w1203, "Row Index"=w1200, "Table reference Array"=w1202) -> ("Error Out"=w1201:errorcluster)  [unwired: 7 in]
            n339 = call "FormatTableStyle.vi"("Format Command"=FormatTableStyle_Commands."Colour Row", "Error In"=w1201, "Row Index"=w1189, "Table reference Array"=w1202) -> ("Error Out"=w1193:errorcluster)  [unwired: 7 in]
            n340 = Index Array(array=w1190, index (row)=w1189, index (col)=8 ("disabled index (col)")) -> (element=w1196:string)
            n341 = String To Path(string=w1196) -> (path=w1194:path)
            n342 = call "ImageIO.vi"("Pos_ImageIO_commands"=ImageIO_commands."ReadImage", "Error In"=w1193, "Image File Path"=w1194, "ImageCluster IN"=w1188) -> ("Error Out"=w1192:errorcluster, "Saved Image OUT"=w1191:T7)  [unwired: 5 in, 1 out]
          }
        }
        n343 = call "GenerateDisplayData.vi"("Index"=w1156, "Error In"=w1159, "UI Controls Refnum"=w1154, "2D Data IN"=w1158) -> ("Error Out"=w1155:errorcluster, "Plot Data OUT"=w1157:cluster{dbl[], dbl[]}[])  [unwired: 4 in, 2 out]
      }
      event "Notes_Table": Mouse Up {
        w1218 = T12 {"CurrentImage"=refnum, "SavedImage"=refnum}  # Image Input Cluster
        # "Did user click on a row within the data range?"
        n344 = event-data() -> ()  [unwired: 1 in, 1 out]
        n345 = Unbundle By Name(w1206) -> ("Big Table"=w1224:refnum<vi>, "Notes Table"=w1212:refnum<vi>)
        n346 = Array Size(array=w1208) -> (size(s)=w1222:i32[])
        n347 = Index Array(array=w1222, index=0) -> (element=w1221:i32)
        n348 = Bundle By Name(cluster=w1218, "SavedImage"=w1217, "CurrentImage"=w1216) -> (w1215:T12)
        n349 = Decrement(x=w1221) -> (x-1=w1229:i32)
        n350 = property class="Tbl (strict)"(reference=w1212, error in=w1231) -> (reference out=w1226:refnum<vi>, error out=w1227:errorcluster, "Selection Start"=w1230:T23)
        n351 = Build Array(w1224, w1212) -> (w1223:refnum<vi>[])
        n352 = Close Reference(reference=w1226, error in (no error)=w1227) -> (error out=w1225:errorcluster)
        n353 = Unbundle By Name(w1230) -> ("Row"=w1220:i32)
        n354 = Less Or Equal?(x=w1220, y=w1229) -> (x <= y?=w1219:bool)
        n355 = case shown="True" w1219 {
          tunnel: w1220 -> [_ w1241]
          tunnel: w1228 -> [w1239 w1252]
          tunnel: [w1239 w1241] -> w1211
          tunnel: w1225 -> [w1238 w1255]
          tunnel: w1223 -> [_ w1254]
          tunnel: [w1238 w1244] -> w1210
          tunnel: [w1236 w1243] -> w1214
          tunnel: w1208 -> [_ w1242]
          tunnel: w1215 -> [w1237 w1240]
          frame False {
            n356 = Unbundle By Name(w1237) -> ("SavedImage"=w1236:T7)
          }
          frame True {
            # "Update index, and highlight\ntable"
            n357 = call "FormatTableStyle.vi"("Format Command"=FormatTableStyle_Commands."Uncolour Row", "Error In"=w1255, "Row Index"=w1252, "Table reference Array"=w1254) -> ("Error Out"=w1253:errorcluster)  [unwired: 7 in]
            n358 = call "FormatTableStyle.vi"("Format Command"=FormatTableStyle_Commands."Colour Row", "Error In"=w1253, "Row Index"=w1241, "Table reference Array"=w1254) -> ("Error Out"=w1245:errorcluster)  [unwired: 7 in]
            n359 = Index Array(array=w1242, index (row)=w1241, index (col)=8 ("disabled index (col)")) -> (element=w1248:string)
            n360 = String To Path(string=w1248) -> (path=w1246:path)
            n361 = call "ImageIO.vi"("Pos_ImageIO_commands"=ImageIO_commands."ReadImage", "Error In"=w1245, "Image File Path"=w1246, "ImageCluster IN"=w1240) -> ("Error Out"=w1244:errorcluster, "Saved Image OUT"=w1243:T7)  [unwired: 5 in, 1 out]
          }
        }
        n362 = call "GenerateDisplayData.vi"("Index"=w1211, "Error In"=w1210, "UI Controls Refnum"=w1206, "2D Data IN"=w1208) -> ("Error Out"=w1209:errorcluster, "Plot Data OUT"=w1207:cluster{dbl[], dbl[]}[])  [unwired: 4 in, 2 out]
      }
      event "Big_Table": Value Change {
        # "Dont allow user to manually change the vallues in the 'BIG Table'; roll back changes if \nany attempts are made.\nThis is done instead of disabling to alow greater user interactivity with teh table through\nselection (allowing user to click on columns anywhere in the table and taking appropriate action)"
        n363 = event-data() -> ("OldVal"=w1280:string[][])  [unwired: 1 in]
        n364 = call "Register_Unregister_UserEvents_PSMGUI.vi"("Event Registration Refnum IN"=w1268, "Action"=enum16{"Register", "Un-Register"}."Un-Register", "error in (no error)"=w1271) -> ("Event Registration Refnum OUT"=w1265:refnum<event-registration>, "error out"=w1269:errorcluster)  [unwired: 8 in, 3 out]
        n365 = Unbundle By Name(w1282) -> ("Big Table"=w1281:refnum<vi>)
        n366 = property class="Tbl (strict)"(reference=w1281, error in=w1269, "Value"=w1280) -> (reference out=w1278:refnum<vi>, error out=w1279:errorcluster)
        n367 = Close Reference(reference=w1278, error in (no error)=w1279) -> (error out=w1267:errorcluster)
        n368 = flat-sequence {
          tunnel: w1267 -> [w1285]
          tunnel: [w1285] -> w1266
          frame #0 {
            n369 = call "Dialog_CannotEdit_Error.vi"() -> ()  [unwired: 12 in]
          }
        }
        n370 = call "Register_Unregister_UserEvents_PSMGUI.vi"("Event Registration Refnum IN"=w1265, "Action"=enum16{"Register", "Un-Register"}."Register", "Pos X IN"=w1262, "Pos Y IN"=w1261, "Pos Z IN"=w1260, "error in (no error)"=w1266) -> ("Event Registration Refnum OUT"=w1263:refnum<event-registration>, "Pos X OUT"=w1259:dbl, "Pos Y OUT"=w1258:dbl, "Pos Z  OUT"=w1257:dbl, "error out"=w1264:errorcluster)  [unwired: 5 in]
      }
      event "Notes_Table": Value Change {
        # "Is selection within range?"
        # "are there any rows?"
        n371 = event-data() -> ("NewVal"=w1316:string[][])  [unwired: 1 in]
        n372 = call "Register_Unregister_UserEvents_PSMGUI.vi"("Event Registration Refnum IN"=w1299, "Action"=enum16{"Register", "Un-Register"}."Un-Register", "Pos X IN"=w1294, "Pos Y IN"=w1293, "Pos Z IN"=w1292, "error in (no error)"=w1300) -> ("Event Registration Refnum OUT"=w1295:refnum<event-registration>, "error out"=w1298:errorcluster)  [unwired: 5 in, 3 out]
        n373 = Array Size(array=w1315) -> (size(s)=w1314:i32[])
        n374 = Index Array(array=w1314, index=0) -> (element=w1308:i32)
        n375 = Increment(x=w1303) -> (x+1=w1309:i32)
        n376 = Greater?(x=w1308, y=0) -> (0:w1307:bool)
        n377 = Less Or Equal?(x=w1309, y=w1308) -> (x <= y?=w1306:bool)
        n378 = And(x=w1306, y=w1307) -> (x .and. y?=w1305:bool)
        n379 = case shown="True" w1305 {
          tunnel: w1298 -> [w1326 w1344]
          tunnel: [w1327 w1333] -> w1317
          tunnel: w1315 -> [w1327 w1343]
          tunnel: w1316 -> [_ w1342]
          tunnel: [w1323 w1335] -> w1296
          tunnel: w1304 -> [w1321 w1336]
          tunnel: w1303 -> [_ w1334]
          frame False {
            # "Discard changes"
            n380 = Unbundle By Name(w1321) -> ("Notes Table"=w1320:refnum<vi>)
            n381 = property class="Tbl (strict)"(reference=w1320, error in=w1326, "Value"=string[][] []) -> (reference out=w1322:refnum<vi>, error out=w1324:errorcluster)
            n382 = Close Reference(reference=w1322, error in (no error)=w1324) -> (error out=w1323:errorcluster)
          }
          frame True {
            # "Update Table UI"
            # "modify notes field"
            # "get new notes"
            # "Write notes to File.\nIf failed, donot update"
            n383 = Index Array(array=w1342, index (col)=0 ("disabled index (col)")) -> (element=w1339:string[])  [unwired: 1 in]
            n384 = Replace Array Subset(array=w1343, new element=w1339, index (col)=7 ("disabled index (col)")) -> (w1338:string[][])  [unwired: 1 in]
            n385 = call "PositionSaveFGV.vi"("PositionSave Commands"=PositionSaveFGVCommands."UpdateEntireTable", "Error In"=w1344, "CompleteTableString"=w1338) -> ("Error Out"=w1337:errorcluster, "Position Data Out"=w1333:string[][])  [unwired: 4 in, 3 out]
            n386 = call "GenerateDisplayData.vi"("Index"=w1334, "Error In"=w1337, "UI Controls Refnum"=w1336, "2D Data IN"=w1333) -> ("Error Out"=w1332:errorcluster, "Notes"=w1331:string[][])  [unwired: 4 in, 2 out]
            n387 = Unbundle By Name(w1336) -> ("Notes Table"=w1330:refnum<vi>)
            n388 = property class="Tbl (strict)"(reference=w1330, error in=w1332, "Value"=w1331) -> (reference out=w1328:refnum<vi>, error out=w1329:errorcluster)
            n389 = Close Reference(reference=w1328, error in (no error)=w1329) -> (error out=w1335:errorcluster)
          }
        }
        n390 = call "Register_Unregister_UserEvents_PSMGUI.vi"("Event Registration Refnum IN"=w1295, "Action"=enum16{"Register", "Un-Register"}."Register", "Pos X IN"=w1294, "Pos Y IN"=w1293, "Pos Z IN"=w1292, "error in (no error)"=w1296) -> ("Event Registration Refnum OUT"=w1291:refnum<event-registration>, "Pos X OUT"=w1290:dbl, "Pos Y OUT"=w1288:dbl, "Pos Z  OUT"=w1287:dbl, "error out"=w1289:errorcluster)  [unwired: 5 in]
      }
      event "Table Navigation Cluster.Table Index Down": Value Change {
        # "No of rows"
        n391 = event-data() -> ()  [unwired: 1 in, 1 out]
        n392 = Unbundle By Name(w1349) -> ("Big Table"=w1368:refnum<vi>, "Notes Table"=w1367:refnum<vi>)
        n393 = Array Size(array=w1351) -> (size(s)=w1364:i32[])
        n394 = Bundle By Name(cluster=T12 {"CurrentImage"=refnum, "SavedImage"=refnum} ("Image Input Cluster"), "SavedImage"=w1358, "CurrentImage"=w1357) -> (w1356:T12)
        n395 = Index Array(array=w1364, index=0) -> (element=w1361:i32)
        n396 = Build Array(w1368, w1367) -> (w1366:refnum<vi>[])
        n397 = Decrement(x=w1361) -> (x-1=w1360:i32)
        n398 = Less?(x=w1362, y=w1360) -> (x < y?=w1369:bool)
        n399 = case shown="True" w1369 {
          tunnel: w1362 -> [w1376 w1394]
          tunnel: [w1376 w1385] -> w1353
          tunnel: w1366 -> [_ w1387]
          tunnel: w1365 -> [w1375 w1393]
          tunnel: [w1375 w1378] -> w1352
          tunnel: w1356 -> [w1374 w1380]
          tunnel: w1351 -> [_ w1386]
          tunnel: [w1373 w1377] -> w1355
          frame False {
            n400 = Unbundle By Name(w1374) -> ("SavedImage"=w1373:T7)
          }
          frame True {
            n401 = call "FormatTableStyle.vi"("Format Command"=FormatTableStyle_Commands."Uncolour Row", "Error In"=w1393, "Row Index"=w1394, "Table reference Array"=w1387) -> ("Error Out"=w1392:errorcluster)  [unwired: 7 in]
            n402 = Increment(x=w1394) -> (x+1=w1385:i32)
            n403 = call "FormatTableStyle.vi"("Format Command"=FormatTableStyle_Commands."Colour Row", "Error In"=w1392, "Row Index"=w1385, "Table reference Array"=w1387) -> ("Error Out"=w1388:errorcluster)  [unwired: 7 in]
            n404 = call "FormatTableStyle.vi"("Format Command"=FormatTableStyle_Commands."UpdateVisibleRows", "Error In"=w1388, "Row Index"=w1385, "Table reference Array"=w1387) -> ("Error Out"=w1379:errorcluster)  [unwired: 7 in]
            n405 = Index Array(array=w1386, index (row)=w1385, index (col)=8 ("disabled index (col)")) -> (element=w1383:string)
            n406 = String To Path(string=w1383) -> (path=w1381:path)
            n407 = call "ImageIO.vi"("Pos_ImageIO_commands"=ImageIO_commands."ReadImage", "Error In"=w1379, "Image File Path"=w1381, "ImageCluster IN"=w1380) -> ("Error Out"=w1378:errorcluster, "Saved Image OUT"=w1377:T7)  [unwired: 5 in, 1 out]
          }
        }
        n408 = call "GenerateDisplayData.vi"("Index"=w1353, "Error In"=w1352, "UI Controls Refnum"=w1349, "2D Data IN"=w1351) -> ("Error Out"=w1350:errorcluster, "Plot Data OUT"=w1348:cluster{dbl[], dbl[]}[])  [unwired: 4 in, 2 out]
      }
      event "Table Navigation Cluster.Table Index Down-End": Value Change {
        # "No of rows > 1?"
        n409 = event-data() -> ()  [unwired: 1 in, 1 out]
        n410 = Unbundle By Name(w1398) -> ("Big Table"=w1418:refnum<vi>, "Notes Table"=w1417:refnum<vi>)
        n411 = Bundle By Name(cluster=T12 {"CurrentImage"=refnum, "SavedImage"=refnum} ("Image Input Cluster"), "SavedImage"=w1407, "CurrentImage"=w1406) -> (w1405:T12)
        n412 = Array Size(array=w1399) -> (size(s)=w1416:i32[])
        n413 = Index Array(array=w1416, index=0) -> (element=w1410:i32)
        n414 = Build Array(w1418, w1417) -> (w1412:refnum<vi>[])
        n415 = Greater?(x=w1410, y=1) -> (0:w1411:bool)
        n416 = case shown="True" w1411 {
          tunnel: w1410 -> [w1424 w1444]
          tunnel: w1414 -> [w1425 w1440]
          tunnel: w1413 -> [_ w1439]
          tunnel: w1412 -> [_ w1438]
          tunnel: [w1425 w1427] -> w1402
          tunnel: [w1424 w1430] -> w1400
          tunnel: w1399 -> [_ w1431]
          tunnel: w1405 -> [w1423 w1428]
          tunnel: [w1422 w1426] -> w1404
          frame False {
            n417 = Unbundle By Name(w1423) -> ("SavedImage"=w1422:T7)
          }
          frame True {
            n418 = call "FormatTableStyle.vi"("Format Command"=FormatTableStyle_Commands."Uncolour Row", "Error In"=w1440, "Row Index"=w1439, "Table reference Array"=w1438) -> ("Error Out"=w1441:errorcluster)  [unwired: 7 in]
            n419 = Decrement(x=w1444) -> (x-1=w1430:i32)
            n420 = call "FormatTableStyle.vi"("Format Command"=FormatTableStyle_Commands."Colour Row", "Error In"=w1441, "Row Index"=w1430, "Table reference Array"=w1438) -> ("Error Out"=w1437:errorcluster)  [unwired: 7 in]
            n421 = call "FormatTableStyle.vi"("Format Command"=FormatTableStyle_Commands."UpdateVisibleRows", "Error In"=w1437, "Row Index"=w1430, "Table reference Array"=w1438) -> ("Error Out"=w1429:errorcluster)  [unwired: 7 in]
            n422 = Index Array(array=w1431, index (row)=w1430, index (col)=8 ("disabled index (col)")) -> (element=w1434:string)
            n423 = String To Path(string=w1434) -> (path=w1432:path)
            n424 = call "ImageIO.vi"("Pos_ImageIO_commands"=ImageIO_commands."ReadImage", "Error In"=w1429, "Image File Path"=w1432, "ImageCluster IN"=w1428) -> ("Error Out"=w1427:errorcluster, "Saved Image OUT"=w1426:T7)  [unwired: 5 in, 1 out]
          }
        }
        n425 = call "GenerateDisplayData.vi"("Index"=w1400, "Error In"=w1402, "UI Controls Refnum"=w1398, "2D Data IN"=w1399) -> ("Error Out"=w1401:errorcluster, "Plot Data OUT"=w1397:cluster{dbl[], dbl[]}[])  [unwired: 4 in, 2 out]
      }
      event "Table Navigation Cluster.Table Index Up-End": Value Change {
        w1458 = T12 {"CurrentImage"=refnum, "SavedImage"=refnum}  # Image Input Cluster
        # "Is no of rows > 1?"
        n426 = event-data() -> ()  [unwired: 1 in, 1 out]
        n427 = Unbundle By Name(w1450) -> ("Big Table"=w1468:refnum<vi>, "Notes Table"=w1467:refnum<vi>)
        n428 = Array Size(array=w1451) -> (size(s)=w1463:i32[])
        n429 = Bundle By Name(cluster=w1458, "SavedImage"=w1457, "CurrentImage"=w1447) -> (w1456:T12)
        n430 = Index Array(array=w1463, index=0) -> (element=w1461:i32)
        n431 = Build Array(w1468, w1467) -> (w1464:refnum<vi>[])
        n432 = Greater?(x=w1461, y=1) -> (0:w1460:bool)
        n433 = case shown="False" w1460 {
          tunnel: w1466 -> [w1475 w1490]
          tunnel: w1465 -> [w1474 w1489]
          tunnel: w1464 -> [_ w1486]
          tunnel: [w1474 w1480] -> w1452
          tunnel: [w1475 w1481] -> w1454
          tunnel: w1451 -> [_ w1479]
          tunnel: w1456 -> [w1473 w1477]
          tunnel: [w1472 w1476] -> w1448
          frame False {
            n434 = Unbundle By Name(w1473) -> ("SavedImage"=w1472:T7)
          }
          frame True {
            w1480 = 0
            n435 = call "FormatTableStyle.vi"("Format Command"=FormatTableStyle_Commands."Uncolour Row", "Error In"=w1490, "Row Index"=w1489, "Table reference Array"=w1486) -> ("Error Out"=w1491:errorcluster)  [unwired: 7 in]
            n436 = call "FormatTableStyle.vi"("Format Command"=FormatTableStyle_Commands."Colour Row", "Error In"=w1491, "Row Index"=w1480, "Table reference Array"=w1486) -> ("Error Out"=w1488:errorcluster)  [unwired: 7 in]
            n437 = call "FormatTableStyle.vi"("Format Command"=FormatTableStyle_Commands."UpdateVisibleRows", "Error In"=w1488, "Row Index"=w1480, "Table reference Array"=w1486) -> ("Error Out"=w1478:errorcluster)  [unwired: 7 in]
            n438 = Index Array(array=w1479, index (row)=w1480, index (col)=8 ("disabled index (col)")) -> (element=w1484:string)
            n439 = String To Path(string=w1484) -> (path=w1482:path)
            n440 = call "ImageIO.vi"("Pos_ImageIO_commands"=ImageIO_commands."ReadImage", "Error In"=w1478, "Image File Path"=w1482, "ImageCluster IN"=w1477) -> ("Error Out"=w1481:errorcluster, "Saved Image OUT"=w1476:T7)  [unwired: 5 in, 1 out]
          }
        }
        n441 = call "GenerateDisplayData.vi"("Index"=w1452, "Error In"=w1454, "UI Controls Refnum"=w1450, "2D Data IN"=w1451) -> ("Error Out"=w1453:errorcluster, "Plot Data OUT"=w1449:cluster{dbl[], dbl[]}[])  [unwired: 4 in, 2 out]
      }
      event "Table Navigation Cluster.Table Index Up": Value Change {
        w1507 = T12 {"CurrentImage"=refnum, "SavedImage"=refnum}  # Image Input Cluster
        n442 = event-data() -> ()  [unwired: 1 in, 1 out]
        n443 = Bundle By Name(cluster=w1507, "SavedImage"=w1506, "CurrentImage"=w1505) -> (w1504:T12)
        n444 = Unbundle By Name(w1497) -> ("Big Table"=w1512:refnum<vi>, "Notes Table"=w1511:refnum<vi>)
        n445 = Build Array(w1512, w1511) -> (w1510:refnum<vi>[])
        n446 = Greater Than 0?(x=w1508) -> (x > 0?=w1513:bool)
        n447 = case shown="False" w1513 {
          tunnel: w1508 -> [w1520 w1538]
          tunnel: [w1520 w1522] -> w1499
          tunnel: w1510 -> [_ w1531]
          tunnel: w1509 -> [w1519 w1537]
          tunnel: [w1519 w1526] -> w1501
          tunnel: w1504 -> [w1518 w1524]
          tunnel: w1498 -> [_ w1523]
          tunnel: [w1517 w1521] -> w1503
          frame False {
            n448 = Unbundle By Name(w1518) -> ("SavedImage"=w1517:T7)
          }
          frame True {
            n449 = call "FormatTableStyle.vi"("Format Command"=FormatTableStyle_Commands."Uncolour Row", "Error In"=w1537, "Row Index"=w1538, "Table reference Array"=w1531) -> ("Error Out"=w1536:errorcluster)  [unwired: 7 in]
            n450 = Decrement(x=w1538) -> (x-1=w1522:i32)
            n451 = call "FormatTableStyle.vi"("Format Command"=FormatTableStyle_Commands."Colour Row", "Error In"=w1536, "Row Index"=w1522, "Table reference Array"=w1531) -> ("Error Out"=w1533:errorcluster)  [unwired: 7 in]
            n452 = call "FormatTableStyle.vi"("Format Command"=FormatTableStyle_Commands."UpdateVisibleRows", "Error In"=w1533, "Row Index"=w1522, "Table reference Array"=w1531) -> ("Error Out"=w1525:errorcluster)  [unwired: 7 in]
            n453 = Index Array(array=w1523, index (row)=w1522, index (col)=8 ("disabled index (col)")) -> (element=w1529:string)
            n454 = String To Path(string=w1529) -> (path=w1527:path)
            n455 = call "ImageIO.vi"("Pos_ImageIO_commands"=ImageIO_commands."ReadImage", "Error In"=w1525, "Image File Path"=w1527, "ImageCluster IN"=w1524) -> ("Error Out"=w1526:errorcluster, "Saved Image OUT"=w1521:T7)  [unwired: 5 in, 1 out]
          }
        }
        n456 = call "GenerateDisplayData.vi"("Index"=w1499, "Error In"=w1501, "UI Controls Refnum"=w1497, "2D Data IN"=w1498) -> ("Error Out"=w1500:errorcluster, "Plot Data OUT"=w1496:cluster{dbl[], dbl[]}[])  [unwired: 4 in, 2 out]
      }
      event Value Change {
        # "Set the Main Image panel\n(EITHER reso or galvo), depending on\nthe system in use"
        # "Typecast to int to make it compatible\nwith both tab types (galvo and reso)"
        # "On user selecting a different channel,\nset the channel no variable to trigger\nthe user event case which refreshes\ncurrent data"
        n457 = event-data() -> ("NewVal"=w1556:T5)  [unwired: 1 in]
        n458 = call "Chnl_2_tab.vi"("Command"=Chnl_2_tab_Commands."ChannelToTab", "Error In"=w1558, "Channel IN"=w1556) -> ("Error Out"=w1557:errorcluster, "Tab Out"=w1547:T16)  [unwired: 6 in, 1 out]
        n459 = Type Cast(type=0 ("x-y 2"), x=w1547) -> (*(type *) &x=w1540:i32)
        n460 = Increment(x=w1540) -> (x+1=w1541:i32)
        n461 = Build Array("MAIN Image panels " ("Variable Name in"), "MAIN Image panels reso " ("Variable Name in")) -> (w1550:string[])
        n462 = for {
          tunnel: w1540 -> [w1572]
          tunnel: w1550 -> [w1569] mode=indexing
          shift-right: [w1571] -> w1545
          shift-left: w1557 -> [w1570]
          n463 = call "GFG_core.vi"("Variable Name in"=w1569, "error in (no error)"=w1570) -> ("Variant Out"=w1568:variant, "error out"=w1565:errorcluster)  [unwired: 11 in, 5 out]
          n464 = Not Equal?(x=variant, y=w1568) -> (x != y?=w1566:bool)
          n465 = case shown="True" w1566 {
            tunnel: w1572 -> [_ w1577]
            tunnel: [w1573 w1576] -> w1571
            tunnel: w1569 -> [_ w1575]
            tunnel: w1565 -> [w1573 w1574]
            frame False {
            }
            frame True {
              n466 = call "GFG_core.vi"("Variable Name in"=w1575, "Variant in"=w1577, "error in (no error)"=w1574, "Action"=enum16{"Init", "Set", "Get"}."Set") -> ("error out"=w1576:errorcluster)  [unwired: 9 in, 6 out]
            }
          }
        }
        n467 = call "GFG_core.vi"("Variable Name in"="channel.no", "Variant in"=w1541, "error in (no error)"=w1545, "Action"=enum16{"Init", "Set", "Get"}."Set") -> ("error out"=w1544:errorcluster)  [unwired: 9 in, 6 out]
      }
      event "step.size.xy 2": Value Change {
        n468 = event-data() -> ("NewVal"=w1590:u16)  [unwired: 1 in]
        n469 = To Variant(anything=w1590) -> (Variant=w1589:variant)
        n470 = call "GFG_core.vi"("Variable Name in"="step.size.xy", "Variant in"=w1589, "error in (no error)"=w1587, "Action"=enum16{"Init", "Set", "Get"}."Set") -> ("error out"=w1586:errorcluster)  [unwired: 9 in, 6 out]
      }
      event "FOCUS2": Value Change {
        n471 = event-data() -> ("NewVal"=w1602:bool)  [unwired: 1 in]
        n472 = To Variant(anything=w1602) -> (Variant=w1603:variant)
        n473 = call "GFGfpRefGet.vi"("Variable Name in"="FOCUS") -> ("output cluster"=w1605:T22)  [unwired: 9 in, 1 out]
        n474 = Unbundle By Name(w1605) -> ("BooleanRef"=w1604:refnum<vi>)
        n475 = property class="Bool"(reference=w1604, error in=w1601, "Val(Sgnl)"=w1603) -> (reference out=w1599:refnum<vi>, error out=w1600:errorcluster)
        n476 = Close Reference(reference=w1599, error in (no error)=w1600) -> (error out=w1598:errorcluster)
      }
      event Key Down {
        w1630 = T12 {"CurrentImage"=refnum, "SavedImage"=refnum}  # Image Input Cluster
        n477 = event-data() -> ("VKey"=w1631:T24)  [unwired: 1 in]
        n478 = Bundle By Name(cluster=w1630, "CurrentImage"=w1629, "SavedImage"=w1625) -> (w1628:T12)
        n479 = case shown="\"ASCII\", Default" w1631 {
          tunnel: w1622 -> [_ w1646 w1651 w1661 w1669]
          tunnel: w1628 -> [_ w1645 w1650 w1660 w1668]
          tunnel: w1621 -> [_ w1644 w1649 w1659 w1667]
          tunnel: w1627 -> [w1636 w1643 w1654 w1662 w1670]
          tunnel: w1626 -> [w1637 w1642 w1652 w1655 w1665]
          tunnel: [w1638 w1641 w1648 w1656 w1664] -> w1624
          tunnel: [w1637 w1640 w1647 w1657 w1663] -> w1620
          tunnel: [w1636 w1639 w1653 w1658 w1666] -> w1623
          tunnel: w1625 -> [w1638 _ _ _ _]
          frame "ASCII", Default {
          }
          frame "Down", "PageDown" {
            n480 = call "Table Index Down.vi"("Table Index IN"=w1642, "error in (no error)"=w1643, "UI Controls Refnum"=w1644, "Image cluster"=w1645, "Formatted Table Data"=w1646) -> ("error out"=w1639:errorcluster, "Table Index OUT"=w1640:i32, "Saved Image OUT"=w1641:T7)  [unwired: 4 in]
          }
          frame "End" {
            n481 = call "Table Index Down_End.vi"("Table Index IN"=w1652, "error in (no error)"=w1654, "UI Controls Refnum"=w1649, "Image cluster"=w1650, "Formatted Table Data"=w1651) -> ("error out"=w1653:errorcluster, "Table Index OUT"=w1647:i32, "Saved Image OUT"=w1648:T7)  [unwired: 4 in]
          }
          frame "Home" {
            n482 = call "Table Index Up_End.vi"("Table Index IN"=w1655, "error in (no error)"=w1662, "UI Controls Refnum"=w1659, "Image cluster"=w1660, "Formatted Table Data"=w1661) -> ("error out"=w1658:errorcluster, "Table Index OUT"=w1657:i32, "Saved Image OUT"=w1656:T7)  [unwired: 4 in]
          }
          frame "Up", "PageUp" {
            n483 = call "Table Index Up.vi"("Table Index IN"=w1665, "error in (no error)"=w1670, "UI Controls Refnum"=w1667, "Image cluster"=w1668, "Formatted Table Data"=w1669) -> ("error out"=w1666:errorcluster, "Table Index OUT"=w1663:i32, "Saved Image OUT"=w1664:T7)  [unwired: 4 in]
          }
        }
        n484 = call "GenerateDisplayData.vi"("Index"=w1620, "Error In"=w1623, "UI Controls Refnum"=w1621, "2D Data IN"=w1622) -> ("Error Out"=w1619:errorcluster, "Plot Data OUT"=w1618:cluster{dbl[], dbl[]}[])  [unwired: 4 in, 2 out]
      }
      event "Vert_Cluster.GO TO": Value Change {
        # "Set the GFG with the values of\nX, Y and Z in the table"
        n485 = event-data() -> ()  [unwired: 1 in, 1 out]
        n486 = Index Array(array=w1689, index (row) #1=w1686, index (col) #1=0 ("disabled index (col)"), index (row) #2=w1686, index (col) #2=1 ("index (row)"), index (row) #3=w1686, index (col) #3=2 ("disabled index (col)")) -> (element #1=w1684:string, element #2=w1683:string, element #3=w1682:string)
        n487 = Fract/Exp String To Number(string=w1684) -> (number=w1680:dbl)  [unwired: 3 in, 1 out]
        n488 = Fract/Exp String To Number(string=w1683) -> (number=w1679:dbl)  [unwired: 3 in, 1 out]
        n489 = Fract/Exp String To Number(string=w1682) -> (number=w1678:dbl)  [unwired: 3 in, 1 out]
        n490 = Bundle By Name(cluster=T18 {"moveXabs"=0.0, "moveYabs"=0.0, "moveZabs"=0.0} ("output cluster"), "moveXabs"=w1680, "moveYabs"=w1679, "moveZabs"=w1678) -> (w1675:T18)
        n491 = call "GFG_core.vi"("Variable Name in"="moveXYZabs", "Variant in"=w1675, "error in (no error)"=w1673, "Action"=enum16{"Init", "Set", "Get"}."Set") -> ("error out"=w1672:errorcluster)  [unwired: 9 in, 6 out]
      }
      event "step.size.z 2": Value Change {
        n492 = event-data() -> ("NewVal"=w1708:u16)  [unwired: 1 in]
        n493 = To Variant(anything=w1708) -> (Variant=w1707:variant)
        n494 = call "GFG_core.vi"("Variable Name in"="step.size.z", "Variant in"=w1707, "error in (no error)"=w1705, "Action"=enum16{"Init", "Set", "Get"}."Set") -> ("error out"=w1704:errorcluster)  [unwired: 9 in, 6 out]
      }
      event Value Change {
        # "Hide FP on user selection"
        n495 = event-data() -> ("NewVal"=w1722:T2)  [unwired: 1 in]
        n496 = case shown="False" w1722 {
          tunnel: [w1729 w1751] -> w1727
          tunnel: w1723 -> [w1731 w1751]
          frame False {
            n497 = control-ref of="This VI"() -> (w1741:refnum<vi>)
            n498 = disable-structure shown="Enabled" {
              disable-tunnel: w1741 -> [w1745 w1749]
              disable-tunnel: [w1744 w1750] -> w1740
              disable-tunnel: [w1743 w1746] -> w1739
              disable-tunnel: w1731 -> [w1742 w1748]
              frame Disabled {
                n499 = invoke class="VI" method="FP.Close"(reference=w1745, error in=w1742) -> (reference out=w1743:refnum<vi>, error out=w1744:errorcluster)  [unwired: 1 in, 1 out]
              }
              frame Enabled {
                n500 = property class="VI"(reference=w1749, error in=w1748, "FP.State"=T13."Hidden" ("Front Panel Window:State")) -> (reference out=w1746:refnum<vi>, error out=w1750:errorcluster)
              }
            }
            n501 = Close Reference(reference=w1739, error in (no error)=w1740) -> (error out=w1732:errorcluster)
            n502 = call "GFGfpRefGet.vi"("error in (no error)"=w1732, "Variable Name in"="PositionSaveButton") -> ("error out"=w1736:errorcluster, "output cluster"=w1737:T22)  [unwired: 8 in]
            n503 = Unbundle By Name(w1737) -> ("BooleanRef"=w1735:refnum<vi>)
            n504 = property class="Bool"(reference=w1735, error in=w1736, "Value"=FALSE) -> (reference out=w1733:refnum<vi>, error out=w1734:errorcluster)
            n505 = Close Reference(reference=w1733, error in (no error)=w1734) -> (error out=w1729:errorcluster)
          }
          frame True {
          }
        }
      }
      event "no of grid lines 2": Value Change {
        n506 = event-data() -> ()  [unwired: 1 in, 1 out]
        n507 = call "IMAQ Clear Overlay"("Image"=w1760) -> ("Image Out"=w1752:T7)  [unwired: 9 in, 1 out]
        n508 = call "GFG_core.vi"("Variable Name in"="no of grid lines", "Variant in"="no of grid lines 2", "Action"=enum16{"Init", "Set", "Get", "Clear"}."Set") -> ()  [unwired: 10 in, 7 out]
      }
    }
    "XY Graph" <- w113
    "posY 2" <- w123
    "posX 2" <- w114
    "posZ 2" <- w122
    "Current Image" <- w108
    "File Path" <- w115
    n509 = flat-sequence {
      frame #0 {
      }
    }
    n510 = Merge Errors(w103, w112) -> (w111:errorcluster)
    n511 = Bundle By Name(cluster=T12 {"CurrentImage"=refnum, "SavedImage"=refnum} ("Image Input Cluster"), "CurrentImage"=w108, "SavedImage"=w107) -> (w106:T12)
    n512 = Unbundle By Name(w111) -> ("status"=w132:bool)
    n513 = call "ImageOverlay.vi"("RGB_Image"=w105, "Error In"=w103, "Overlay?"="Overlay", "UI Controls Refnum"=w110, "Image Input Cluster"=w106) -> ("Error Out"=w102:errorcluster, "Saved Image"=w99:T7)  [unwired: 5 in]
    n514 = call "grid_overlay and calculate grid size.vi"("Image In"=w99) -> ("Image Out"=→"Saved Image":T7)  [unwired: 10 in]
    n515 = Or(x=w132, y=w133) -> (x .or. y?=w131:bool)
  }
  n516 = Unregister For Events(event registration refnum=w62, error in=w33) -> (error out=w69:errorcluster)
  n517 = call <vilib>:"Simple Error Handler.vi"("error in (no error)"=w69) -> ("error out"=w34:errorcluster)  [unwired: 4 in, 4 out]
  n518 = call <vilib>:"Clear Errors.vi"("error in (no error)"=w34) -> ("error out"=w15:errorcluster)  [unwired: 6 in]
  n519 = call "IMAQ Dispose"("Image"=w13, "error in (no error)"=w15) -> ("error out"=w11:errorcluster)  [unwired: 4 in]
  n520 = call "IMAQ Dispose"("Image"=w12, "error in (no error)"=w11) -> ("error out"=w14:errorcluster)  [unwired: 4 in]
  n521 = call "PositionSaveFGV.vi"("PositionSave Commands"=PositionSaveFGVCommands."Shutdown and Cleanup", "Error In"=w14) -> ()  [unwired: 5 in, 5 out]
